vi "Central_Controller_SEF.vi"() -> ()   [LabVIEW 2019]
uses:
  <vilib>/Modbus/master/Modbus Master.lvclass
  C:/Program Files (x86)/National Instruments/LabVIEW 2019/vi.lib/Modbus/subvis/Modbus API/Modbus API.lvclass
  <vilib>/Modbus/subvis/Modbus API/Modbus API.lvclass/Modbus API.ctl
  <vilib>/Modbus/subvis/Transmission Data Unit (ADU)/Transmission Data Unit/Transmission Data Unit.lvclass/Transmission Data Unit.ctl
  <vilib>/Modbus/master/Data Access/Unit ID/Set Unit ID Property.vi
  <vilib>/Modbus/subvis/Transmission Data Unit (ADU)/Transmission Data Unit/Data Access/Unit ID/Write Unit ID.vi
  <vilib>/Modbus/subvis/Modbus API/Read Transmission Data Unit.vi
  <vilib>/Modbus/subvis/Modbus API/Write Transmission Data Unit.vi
  <vilib>/Modbus/master/Create Master Instance (TCP).vi
  <vilib>/Modbus/subvis/Transmission Data Unit (ADU)/Transmission Data Unit/Transmission Data Unit.lvclass
panel:
  out "Correct":bool
  out "Frequency":sgl
  out "SOLAR Real Power":sgl[](array[numeric])
  out "Array":errorcluster[](array[cluster])
  in  "Tab Control Islanding Extras":enum32{"Page 1"}(tab)
  in  "Relay 1 Num":u16
  in  "Relay 2 Num":u16
  in  "Relay 1":bool
  in  "Relay 2":bool
  in  "Tab Control Optimization Extras":enum32{"Page 1"}(tab)
  out "OPT Price":sgl[](array[numeric]) format="%#.3f"
  in  "OPT Alpha":sgl=0.1
  out "OPT Running No Error":bool
  out "In Range?":bool
  in  "Coerce":bool
  out "Attempts":i32
  in  "Reset Dual Variables":bool
  in  "Dispatch":bool
  in  "Array DER Index Dispatch":bool[](array[boolean])=[TRUE, TRUE, TRUE, TRUE, TRUE, TRUE, TRUE, TRUE, TRUE, TRUE, TRUE, TRUE, TRUE, FALSE, FALSE, TRUE]
  out "Pmax":sgl
  out "Pmin":sgl
  out "Pmin,i":sgl[](array[numeric])
  out "Pmax,i":sgl[](array[numeric])
  out "Indicator 15":sgl[](array[numeric])
  out "Indicator 14":sgl[](array[numeric])
  out "Indicator 13":sgl[](array[numeric])
  out "Indicator 12":sgl[](array[numeric])
  out "Indicator 11":sgl[](array[numeric])
  out "Indicator 10":sgl[](array[numeric])
  out "Indicator 9":sgl[](array[numeric])
  out "Indicator 8":sgl[](array[numeric])
  out "Indicator 7":sgl[](array[numeric])
  out "Indicator 6":sgl[](array[numeric])
  out "Indicator 5":sgl[](array[numeric])
  out "Indicator 4":sgl[](array[numeric])
  out "Indicator 3":sgl[](array[numeric])
  out "Indicator 2":sgl[](array[numeric])
  out "Indicator 1":sgl[](array[numeric])
  out "Indicator 0":sgl[](array[numeric])
  in  "DER List":string[](array[string])=["Capstone", "Aquion", "Tesla", "Load Bank", "Motor 1", "Simpliphi 1", "LG Chem", "Outback 1", "Outback 2", "Sunny Island", "ESS", "Fuel Cells", "Sparkplug", "Fronius", "Suny Boy", "Motor 2"]
  out "data":T1
  in  "File Name":string
  out "error out 3":errorcluster
  in  "Folder":path=path "C:/Users/administrator.STONEEDGEPOWER/Desktop/Data"
  out "Bid":sgl[](array[numeric])
  out "ALL Status":u16[](array[numeric])
  out "ALL AC RMS Line-Neutral Voltages":sgl[][](array[numeric])
  out "SYS Current Time":dbl format="%.3f"
  out "SYS DER Index":i32
  out "ALL Frequency":sgl[](array[numeric])
  out "ALL Control Method":string[](array[string])
  out "ALL Logged":bool[](array[boolean])
  out "ALL Through Variable":sgl[](array[numeric])
  out "ALL Across Variable":sgl[](array[numeric])
  out "ALL State of Charge":sgl[](array[numeric])
  out "ALL Reactive Power":sgl[](array[numeric])
  out "ALL Real Power":sgl[](array[numeric])
  out "ALL AC RMS Line-Line Average Voltage":sgl[][](array[numeric])
  in  "Tab Control Main":T2(tab)
  out "SYS H2 SoC":sgl format="%.1f"
  out "SYS H2 SoC Figure":sgl(slide) scale=0.0..100.0
  out "Free Power Flow Plot":sgl(graph)
  out "Free Power Flow Gauge":sgl(knob) caption="Gauge" scale=-100.0..100.0
  out "SYS SoC":sgl format="%.1f"
  out "SYS SoC Figure":sgl(slide) scale=0.0..100.0
  out "Free Power Flow":sgl
  out "DER0 Control Mode":string="Slave Mode Droops"
  out "LOAD Flow":i32(ring)
  out "LOAD Total Real Power":sgl format="%#.1f"
  out "DER13 Power Level":sgl format="%#.1f"
  out "DER14 Power Level":sgl format="%#.1f"
  out "DER13 Power Level Figure":sgl(slide)=1.0 scale=0.0..100.0
  out "DER3 State of Charge Figure":sgl(slide) scale=0.0..100.0
  out "DER3 State of Charge":sgl format="%.1f"
  out "DER0 Power Level Figure":sgl(slide)=1.0 scale=0.0..100.0
  out "DER14 Power Level Figure":sgl(slide)=1.0 scale=0.0..100.0
  out "SOLAR Flow":i32(ring)
  out "SOLAR Total Real Power":sgl format="%#.1f"
  out "DER15 Flow":i32(ring)
  out "DER14 Flow":i32(ring)
  out "DER13 Flow":i32(ring)
  out "DER12 Flow":i32(ring)
  out "DER5 Flow":i32(ring)
  out "DER4 Flow":i32(ring)
  out "DER3 Flow":i32(ring)
  out "DER1 Flow":i32(ring)
  out "DER0 Flow":i32(ring)
  in  "DER15 Detail Window Button":bool
  out "DER9 Reactive Power":sgl format="%.1f"
  out "DER10 State of Charge Figure":sgl(slide) scale=0.0..100.0
  out "DER10 State of Charge":sgl format="%#.1f"
  out "DER10 DC Voltage":sgl format="%.1f"
  out "PCC Meter":string
  in  "DER10 Detail Window Button":bool
  in  "DER13 Detail Window Button":bool
  in  "DER12 Detail Window Button":bool
  in  "DER2 Detail Window Button":bool
  in  "DER5 Detail Window Button":bool
  in  "DER9 Detail Window Button":bool
  in  "DER14 Detail Window Button":bool
  out "DER15 State of Charge Figure":sgl(slide) scale=0.0..100.0
  out "DER15 State of Charge":sgl format="%#.1f"
  out "DER15 Real Power":sgl format="%.1f"
  in  "DER15 Login Button":bool
  out "DER15 Logged":bool
  out "DER15 DC Voltage":sgl format="%#.1f"
  out "DER15 AC Line-Line Voltage":sgl=209.57935 format="%.1f"
  out "DER15 State":string
  in  "Island":bool
  out "DER8 State of Charge Figure":sgl(slide) scale=0.0..100.0
  out "DER8 State of Charge":sgl format="%#.1f"
  out "DER7 State of Charge Figure":sgl(slide) scale=0.0..100.0
  out "DER7 State of Charge":sgl format="%.1f"
  out "DER14 Real Power":sgl format="%.1f"
  in  "DER14 Login Button":bool
  out "DER14 Logged":bool
  out "DER14 DC Voltage":sgl format="%#.1f"
  out "DER14 AC Line-Line Voltage":sgl=209.57935 format="%.1f"
  out "DER9 State of Charge Figure":sgl(slide) scale=0.0..100.0
  out "DER9 Across Variable":sgl format="%.1g"
  out "DER9 State of Charge":sgl format="%.1f"
  out "DER13 AC Line-Line Voltage":sgl format="%.1f"
  out "DER13 Real Power":sgl format="%.1f"
  in  "DER13 Login Button":bool
  out "DER13 Logged":bool
  out "PCC Flow":i32(ring)
  out "DER8 DC Voltage":sgl format="%.1f"
  out "DER10 AC Line-Line Votlage":sgl format="%.1f"
  out "DER10 Real Power":sgl format="%.1f"
  in  "DER10 Login Button":bool
  out "DER10 Logged":bool
  out "DER7 Real Power":sgl format="%.1f"
  out "DER4 AC Line-Line Votlage":sgl format="%.1f"
  out "DER5 State of Charge Figure":sgl(slide) scale=0.0..100.0
  in  "DER0 Login Button":bool
  in  "DER2 Login Button":bool
  in  "DER1 Login Button":bool
  out "DER2 State of Charge Figure":sgl(slide) scale=0.0..100.0
  out "DER1 State of Charge Figure":sgl(slide) scale=0.0..100.0
  out "DER1 Real Power":sgl format="%.1f"
  out "DER1 Reactive Power":sgl format="%#.1f"
  out "DER1 AC Line-Line Voltage":sgl format="%.1f"
  out "DER2 Frequency":sgl format="%.1f"
  out "DER0 Real Power":sgl format="%#.1f"
  out "DER0 AC Line-Line Voltage":sgl format="%#.1f"
  out "DER2 AC Line-Line Voltage":sgl format="%.1f"
  out "DER2 Reactive Power":sgl format="%.1f"
  out "DER2 Real Power":sgl format="%.1f"
  out "DER0 Logged":bool
  out "DER1 Logged":bool
  out "DER2 Logged":bool
  out "DER0 Power Level":sgl format="%#.1f"
  out "DER1 State of Charge":sgl format="%.1f"
  out "DER2 State of Charge":sgl format="%#.1f"
  out "PCC Reactive Power":sgl
  out "PCC Real Power":sgl
  out "PCC AC Line-Line Voltage":sgl format="%#.1f"
  out "PCC Frequency":sgl format="%.2g"
  in  "DER3 Login Button":bool
  out "DER3 Logged":bool
  out "DER3 Real Power":sgl format="%#.1f"
  out "DER3 AC Line-Line Votlage":sgl format="%#.1f"
  out "DER4 State of Charge Figure":sgl(slide) scale=0.0..100.0
  out "DER4 State of Charge":sgl format="%#.1f"
  in  "DER4 Login Button":bool
  out "DER4 Logged":bool
  in  "DER5 Login Button":bool
  out "DER5 Across Variable":sgl format="%#.1f"
  out "DER5 logged":bool
  out "DER5 AC Line-Line Votlage":sgl format="%.1f"
  out "DER5 Real Power":sgl format="%.1f"
  out "PCC Real Power Duplicate":sgl format="%#_4g"
  in  "OPT Microgrid Set-point":sgl
  out "OPT Optimization Running Indicator":bool=TRUE
  in  "OPT Start Button":bool
  in  "OPT Stop Button":bool
  out "DER5 State of Charge":sgl format="%.1f"
  in  "DER7 Login Button":bool
  in  "DER8 Login Button":bool
  in  "DER9 Login Button":bool
  out "DER7 Logged":bool
  out "DER7 DC Voltage":sgl format="%.1g"
  out "DER7 AC Line-Line Voltage":sgl=209.57935 format="%.1f"
  out "DER8 AC Line-Line Votlage":sgl format="%.1f"
  out "DER8 Real Power":sgl format="%.1f"
  out "DER8 Logged":bool
  out "DER9 AC Line-Line Votlage":sgl format="%.1f"
  out "DER9 Real Power":sgl format="%.1f"
  out "DER9 Logged":bool
  out "DER12 AC Line-Line Votlage":sgl=209.57935 format="%.1f"
  out "DER12 DC Voltage":sgl format="%.1g"
  out "DER12 Logged":bool
  in  "DER12 Login Button":bool
  out "DER12 Real Power":sgl format="%.1g"
  out "DER4 Across Variable":sgl format="%#.1f"
  out "DER4 Real Power":sgl format="%#.1f"
  out "DER0 State":string
  out "DER1 State":string
  out "DER2 State":string
  out "DER3 State":string
  out "DER4 State":string
  out "DER5 State":string
  out "DER7 State":string
  out "DER8 State":string
  out "DER9 State":string
  out "DER10 State":string
  out "DER12 State":string
  out "DER13 State":string
  out "DER14 State":string
  in  "Reconnect":bool
  in  "DER0 Control Window Button":bool
  in  "DER0 Detail Window Button":bool
  in  "DER1 Detail Window Button":bool
  in  "DER1 Control Window Button":bool
  in  "DER2 Control Window Button":bool
  in  "DER3 Control Window Button":bool
  in  "DER4 Control Window Button":bool
  in  "DER5 Control Window Button":bool
  in  "DER7 Control Window Button":bool
  in  "DER8 Control Window Button":bool
  in  "DER9 Control Window Button":bool
  in  "DER10 Control Window Button":bool
  in  "DER12 Control Window Button":bool
  in  "DER13 Control Window Button":bool
  in  "DER14 Control Window Button":bool
  in  "DER15 Control Window Button":bool
  out "DER12 State of Charge":sgl format="%#.1f"
  out "DER12 State of Charge Figure":sgl(slide) scale=0.0..100.0
  in  "DER7 Detail Window Button":bool
  in  "DER3 Detail Window Button":bool
  in  "DER4 Detail Window Button":bool
  in  "DER8 Detail Window Button":bool
  out "DER2 Control Mode":string="Slave Mode Droops"
  out "DER14 Reactive Power":sgl format="%.1f"
  out "DER13 Reactive Power":sgl format="%.1f"
  out "DER1 Control Mode":string="Slave Mode Droops"
  out "DER2 Flow":i32(ring)
  out "DER7 Flow":i32(ring)
  out "DER8 Flow":i32(ring)
  out "DER9 Flow":i32(ring)
  out "DER10 Flow":i32(ring)
  out "PCC Real Power Figure":T3(graph)
  out "DER11 Flow":i32(ring)
  in  "DER11 Control Window Button":bool
  out "DER11 State":string
  out "DER11 AC Line-Line Votlage":sgl=209.57935 format="%.1f"
  out "DER11 Logged":bool
  in  "DER11 Login Button":bool
  out "DER11 Real Power":sgl format="%.1f"
  in  "DER11 Detail Window Button":bool
  out "DER11 Reactive Power":sgl format="%.1f"
  out "DER11 State of Charge":sgl format="%.1f"
  out "DER11 State of Charge Figure":sgl(slide) scale=0.0..100.0
  in  "DER6 Control Window Button":bool
  out "DER6 State":string
  out "DER6 AC Line-Line Voltage":sgl format="%.1f"
  out "DER6 Reactive Power":sgl format="%.1g"
  out "DER6 State of Charge":sgl format="%.1f"
  out "DER6 State of Charge Figure":sgl(slide) scale=0.0..100.0
  out "DER Logged":bool
  in  "DER6 Login Button":bool
  out "DER6 Real Power":sgl format="%.1g"
  in  "DER6 Detail Window Button":bool
  out "DER6 Flow":i32(ring)
  in  "Tab Control Communications":enum32{"Page 1"}(tab)
  in  "Enable Array":bool[](array[boolean])=[TRUE, FALSE, TRUE, FALSE, TRUE, TRUE, TRUE, FALSE, TRUE, TRUE, FALSE, FALSE, TRUE, TRUE, TRUE, TRUE]
  out "ALL Error Indicator":bool[](array[boolean])
  out "ALL DER Current Error":errorcluster[](array[cluster])
  out "ALL DER Final Error":errorcluster[](array[cluster])
  in  "PCC Meter IP Address":string[](array[string])=["10.0.1.53", "10.0.1.18"]
  out "PQM Current Error":errorcluster
  out "PQM Final Error":errorcluster
  in  "IP Address List":string[](array[string])=["10.0.1.182", "10.0.1.184", "10.0.1.180", "10.0.1.202", "10.0.1.189", "10.0.1.188", "10.0.1.190", "10.0.1.187", "10.0.1.195", "10.0.1.191", "10.0.1.185", "10.0.1.181", "10.0.1.201", "10.0.1.192", "10.0.1.207", "10.0.1.196"]
  in  "DERs Label Name":string[](array[string])=["DER0", "DER1", "DER2", "DER3", "DER4", "DER5", "DER6", "DER7", "DER8", "DER9", "DER10", "DER11", "DER12", "DER13", "DER14", "DER15"]
  out "Egauge Final Error":errorcluster
  out "Egauge Current Error":errorcluster
  out "SYS Iteration":i32
  in  "stop":bool
  out "SYS Status":string="Reading"
  out "SYS Case":i32
  in  "PCC Meter Label Name":string[](array[string])=["ASCO PQM", "Egauge"]
  in  "Solar Meter IP Address":string[](array[string])=["10.0.1.16"]
  in  "Solar Meter Label Name":string[](array[string])=["Solar 1 (Butler)", "Solar 2 (Agshed)", "Solar 3", "Solar 4", "Solar 5", "Solar 6"]
  out "PCC Meter Error Indicators":bool[](array[boolean])
  out "Solar Meter Error Indicators":bool[](array[boolean])
  # "DER0: Heila 2 , CAPSTONE, .182\nDER1: Heila 4, AQUION, .184\nDER2: Heila 0, TESLA, .180\nDER3: Heila 22, Load Bank, .202\nDER4: Heila 9, MOTOR 1, .189\nDER5: Heila 8, SIMPLIPHI 1, .188\nDER6: Heila 10, Solar Edge, .190\nDER7: Heila 7, OUTBACK 1, .187\nDER8: Heila15, OUTBACK 2, .195\nDER9: Heila 12, SUNNY ISLAND, .191\nDER10: Heila 5, ESS, .185\nDER11: Heila 1, Fuel Cells, .181\nDER12: Heila 21. Sparkplug, .201\nDER13: Heila 12, Fronius, .192\nDER14: Heila 27, Sunny Boy, .207\nDER15: Heila 16, Motor 2, .196"
  # "Islanding Extras"
  # "Optimization Extras"
  # "Consumption"
  # "Generation"
  # "Excess  Consumption"
  # "Excess Generation"
  # "Solar"
  # "Gas Turbine"
  # "HVAC"
  # "Loads"
  # "Battery"
  # "Hydrogen"
  # "SoC"
  # "%"
  # "SoC"
  # "%"
  # "Battery"
  # "Battery"
  # "Motor"
  # "Gas Turbine"
  # "Battery"
  # "Electrolyzer"
  # "Solar"
  # "Motor"
  # "Outback FLEX power"
  # "Capstone"
  # "Aquion + Ideal Power"
  # "Giner"
  # "LG + SolarEdge"
  # "LG + Sunny Boy"
  # "Hitachi VFD"
  # "Hitachi VFD"
  # "Status:"
  # "Status:"
  # "Status:"
  # "Status:"
  # "Status:"
  # "Status:"
  # "Status:"
  # "Status:"
  # "Mode:"
  # "Mode:"
  # "Solar"
  # "V"
  # "psi"
  # "V"
  # "psi"
  # "Real Microgrid in Real Time"
  # "SoC"
  # "%"
  # "SoC"
  # "SoC"
  # "%"
  # "SoC"
  # "%"
  # "p.u."
  # "%"
  # "%"
  # "SoC"
  # "%"
  # "p.u."
  # "%"
  # "SoC"
  # "%"
  # "kW"
  # "kW"
  # "kW"
  # "kW"
  # "kW"
  # "kW"
  # "kW"
  # "kW"
  # "Utility Grid"
  # "kW"
  # "V ="
  # "V"
  # "V"
  # "kVAr"
  # "V"
  # "V"
  # "kVAr"
  # "V"
  # "kVAr"
  # "V"
  # "f ="
  # "Hz"
  # "PG&E"
  # "P ="
  # "W"
  # "V"
  # "V"
  # "V"
  # "Q ="
  # "VAr"
  # "Optimization:"
  # "kW"
  # "kW"
  # "kW"
  # "kVAr"
  # "kW"
  # "kW"
  # "PCC Set-point:"
  # "kW"
  # "kW"
  # "kW"
  # "kW"
  # "V"
  # "kVAr"
  # "kVAr"
  # "kW"
  # "kVAr"
  # "V"
  # "V"
  # "V"
  # "V"
  # "V"
  # "V"
  # "V"
  # "Hz"
  # "PCC Power:"
  # "kW"
  # "Battery"
  # "Battery"
  # "Fuel Cells"
  # "Battery"
  # "Battery"
  # "Battery"
  # "Battery"
  # "Solar"
  # "Load"
  # "Sony + Outback"
  # "Relion"
  # "Simpliphi + SMA"
  # "Tesla + Dynapower"
  # "Simpliphi + Schneider"
  # "Simpliphi + Schneider"
  # "LG + Fronius"
  # "ESS"
  # "Status:"
  # "Status:"
  # "Status:"
  # "Status:"
  # "Status:"
  # "Status:"
  # "Status:"
  # "Status:"
  # "Mode:"
  # "V"
  # "V"
  # "V"
  # "V"
  # "V"
  # "SoC"
  # "%"
  # "SoC"
  # "%"
  # "SoC"
  # "%"
  # "SoC"
  # "%"
  # "SoC"
  # "%"
  # "SoC"
  # "%"
  # "SoC"
  # "%"
  # "p.u."
  # "%"
  # "Reading from:"
  # "Program"
  # "Controllable DERs"
  # "PCC Meters"
  # "Solar Array Meters"
  # "DER0: Heila 2 , CAPSTONE, .182\nDER1: Heila 4, AQUION, .184\nDER2: Heila 0, TESLA, .180\nDER3: Heila 22, Load Bank, .202\nDER4: Heila 9, MOTOR 1, .189\nDER5: Heila 8, SIMPLIPHI 1, .188\nDER6: Heila 10, Solar Edge, .190\nDER7: Heila 7, OUTBACK 1, .187\nDER8: Heila15, OUTBACK 2, .195\nDER9: Heila 12, SUNNY ISLAND, .191\nDER10: Heila 5, ESS, .185\nDER11: Heila 1, Fuel Cells, .181\nDER12: Heila 21. Sparkplug, .201\nDER13: Heila 12, Fronius, .192\nDER14: Heila 27, Sunny Boy, .207\nDER15: Heila 16, Motor 2, .196"
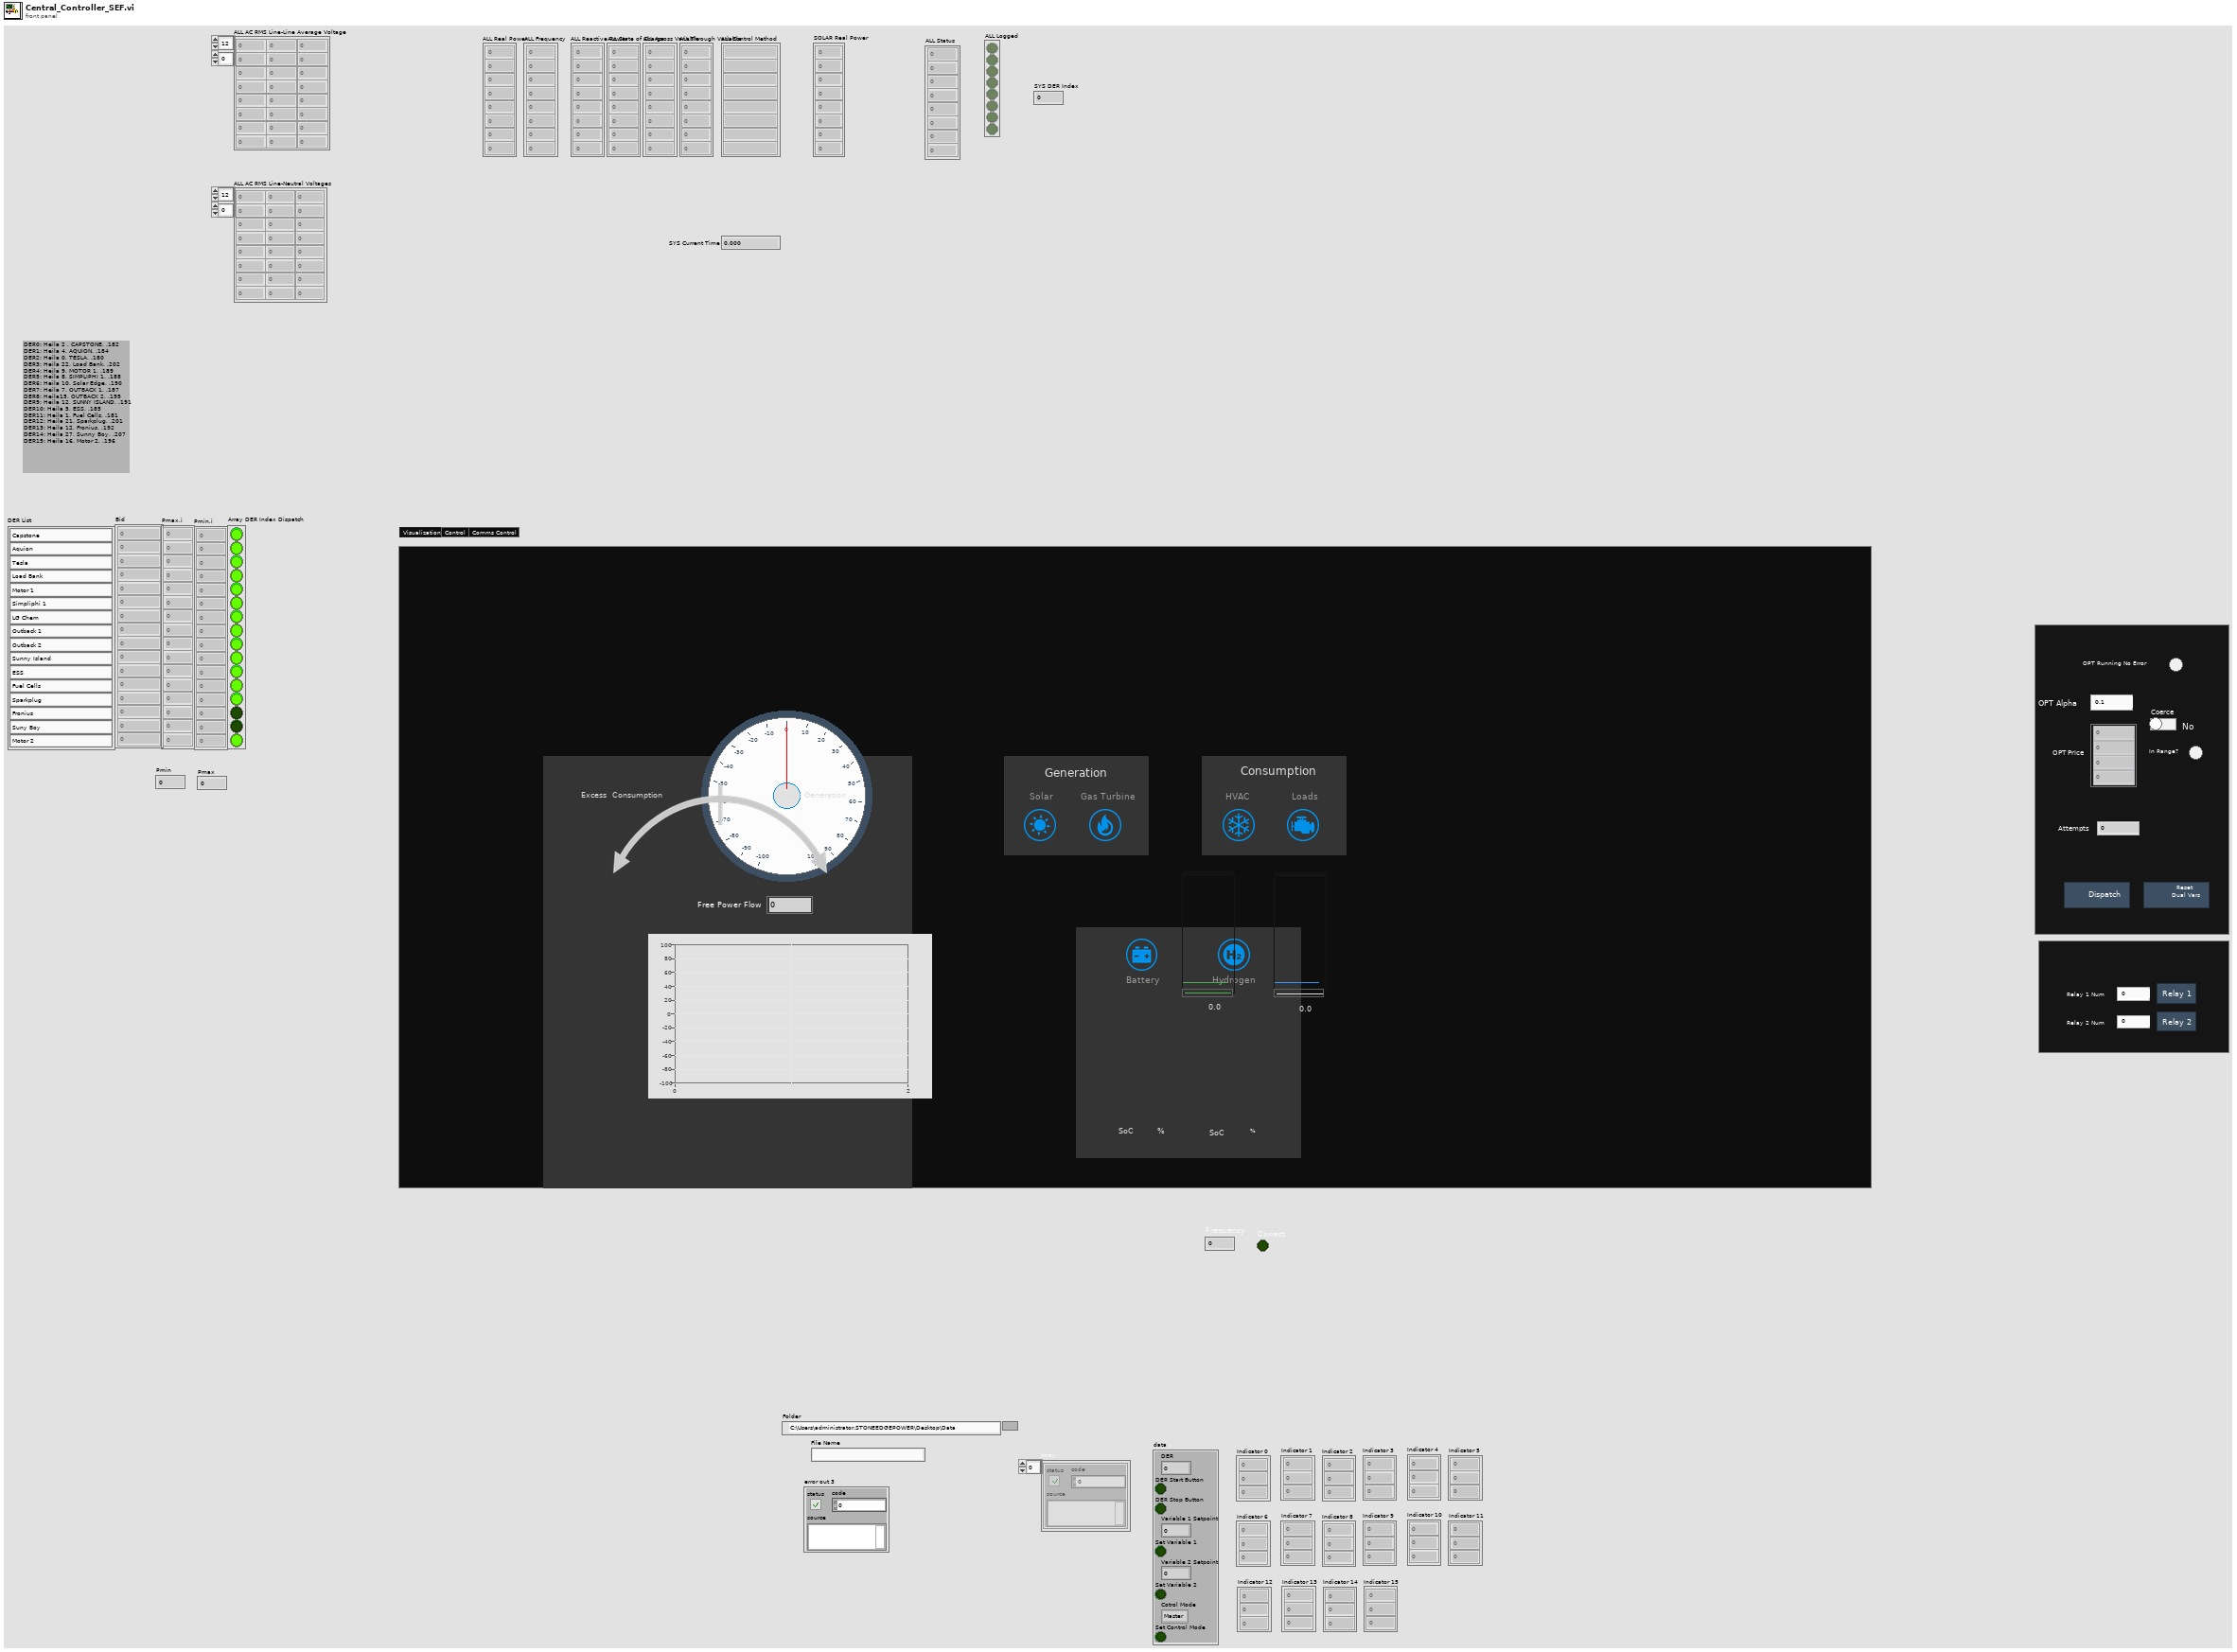
[diagram p1: front panel]
types:
  T1 = cluster{"DER":i32, "DER Start Button":bool, "DER Stop Button":bool, "Variable 1 Setpoint":sgl, "Set Variable 1":bool, "Variable 2 Setpoint":sgl, "Set Variable 2":bool, "Cotrol Mode":enum16{"Master", "Slave"}, "Set Control Mode":bool}
  T2 = enum32{"Visualization", "Control", "Comms Control"}
  T3 = cluster{"[0]":sgl, "[1]":sgl, "[2]":sgl, "[3]":sgl, "[4]":sgl}
  T4 = enum16{"open", "replace", "create", "open or create", "replace or create", "replace or create with confirmation"}
  T5 = cluster{"Modbus master out":refnum<class "Modbus Master.lvclass">, "error out":errorcluster}[]
  T6 = cluster{"Modbus master out":refnum<class "Modbus Master.lvclass">, "error out":errorcluster}
  T7 = enum32{"Invalid", "Standard", "Closed", "Hidden", "Minimized", "Maximized"}
  T8 = cluster{"Modbus master out":refnum<class "Modbus Master.lvclass">, "error IO":errorcluster}
  T9 = enum32{"Bad", "Idle", "Run top level", "Running"}
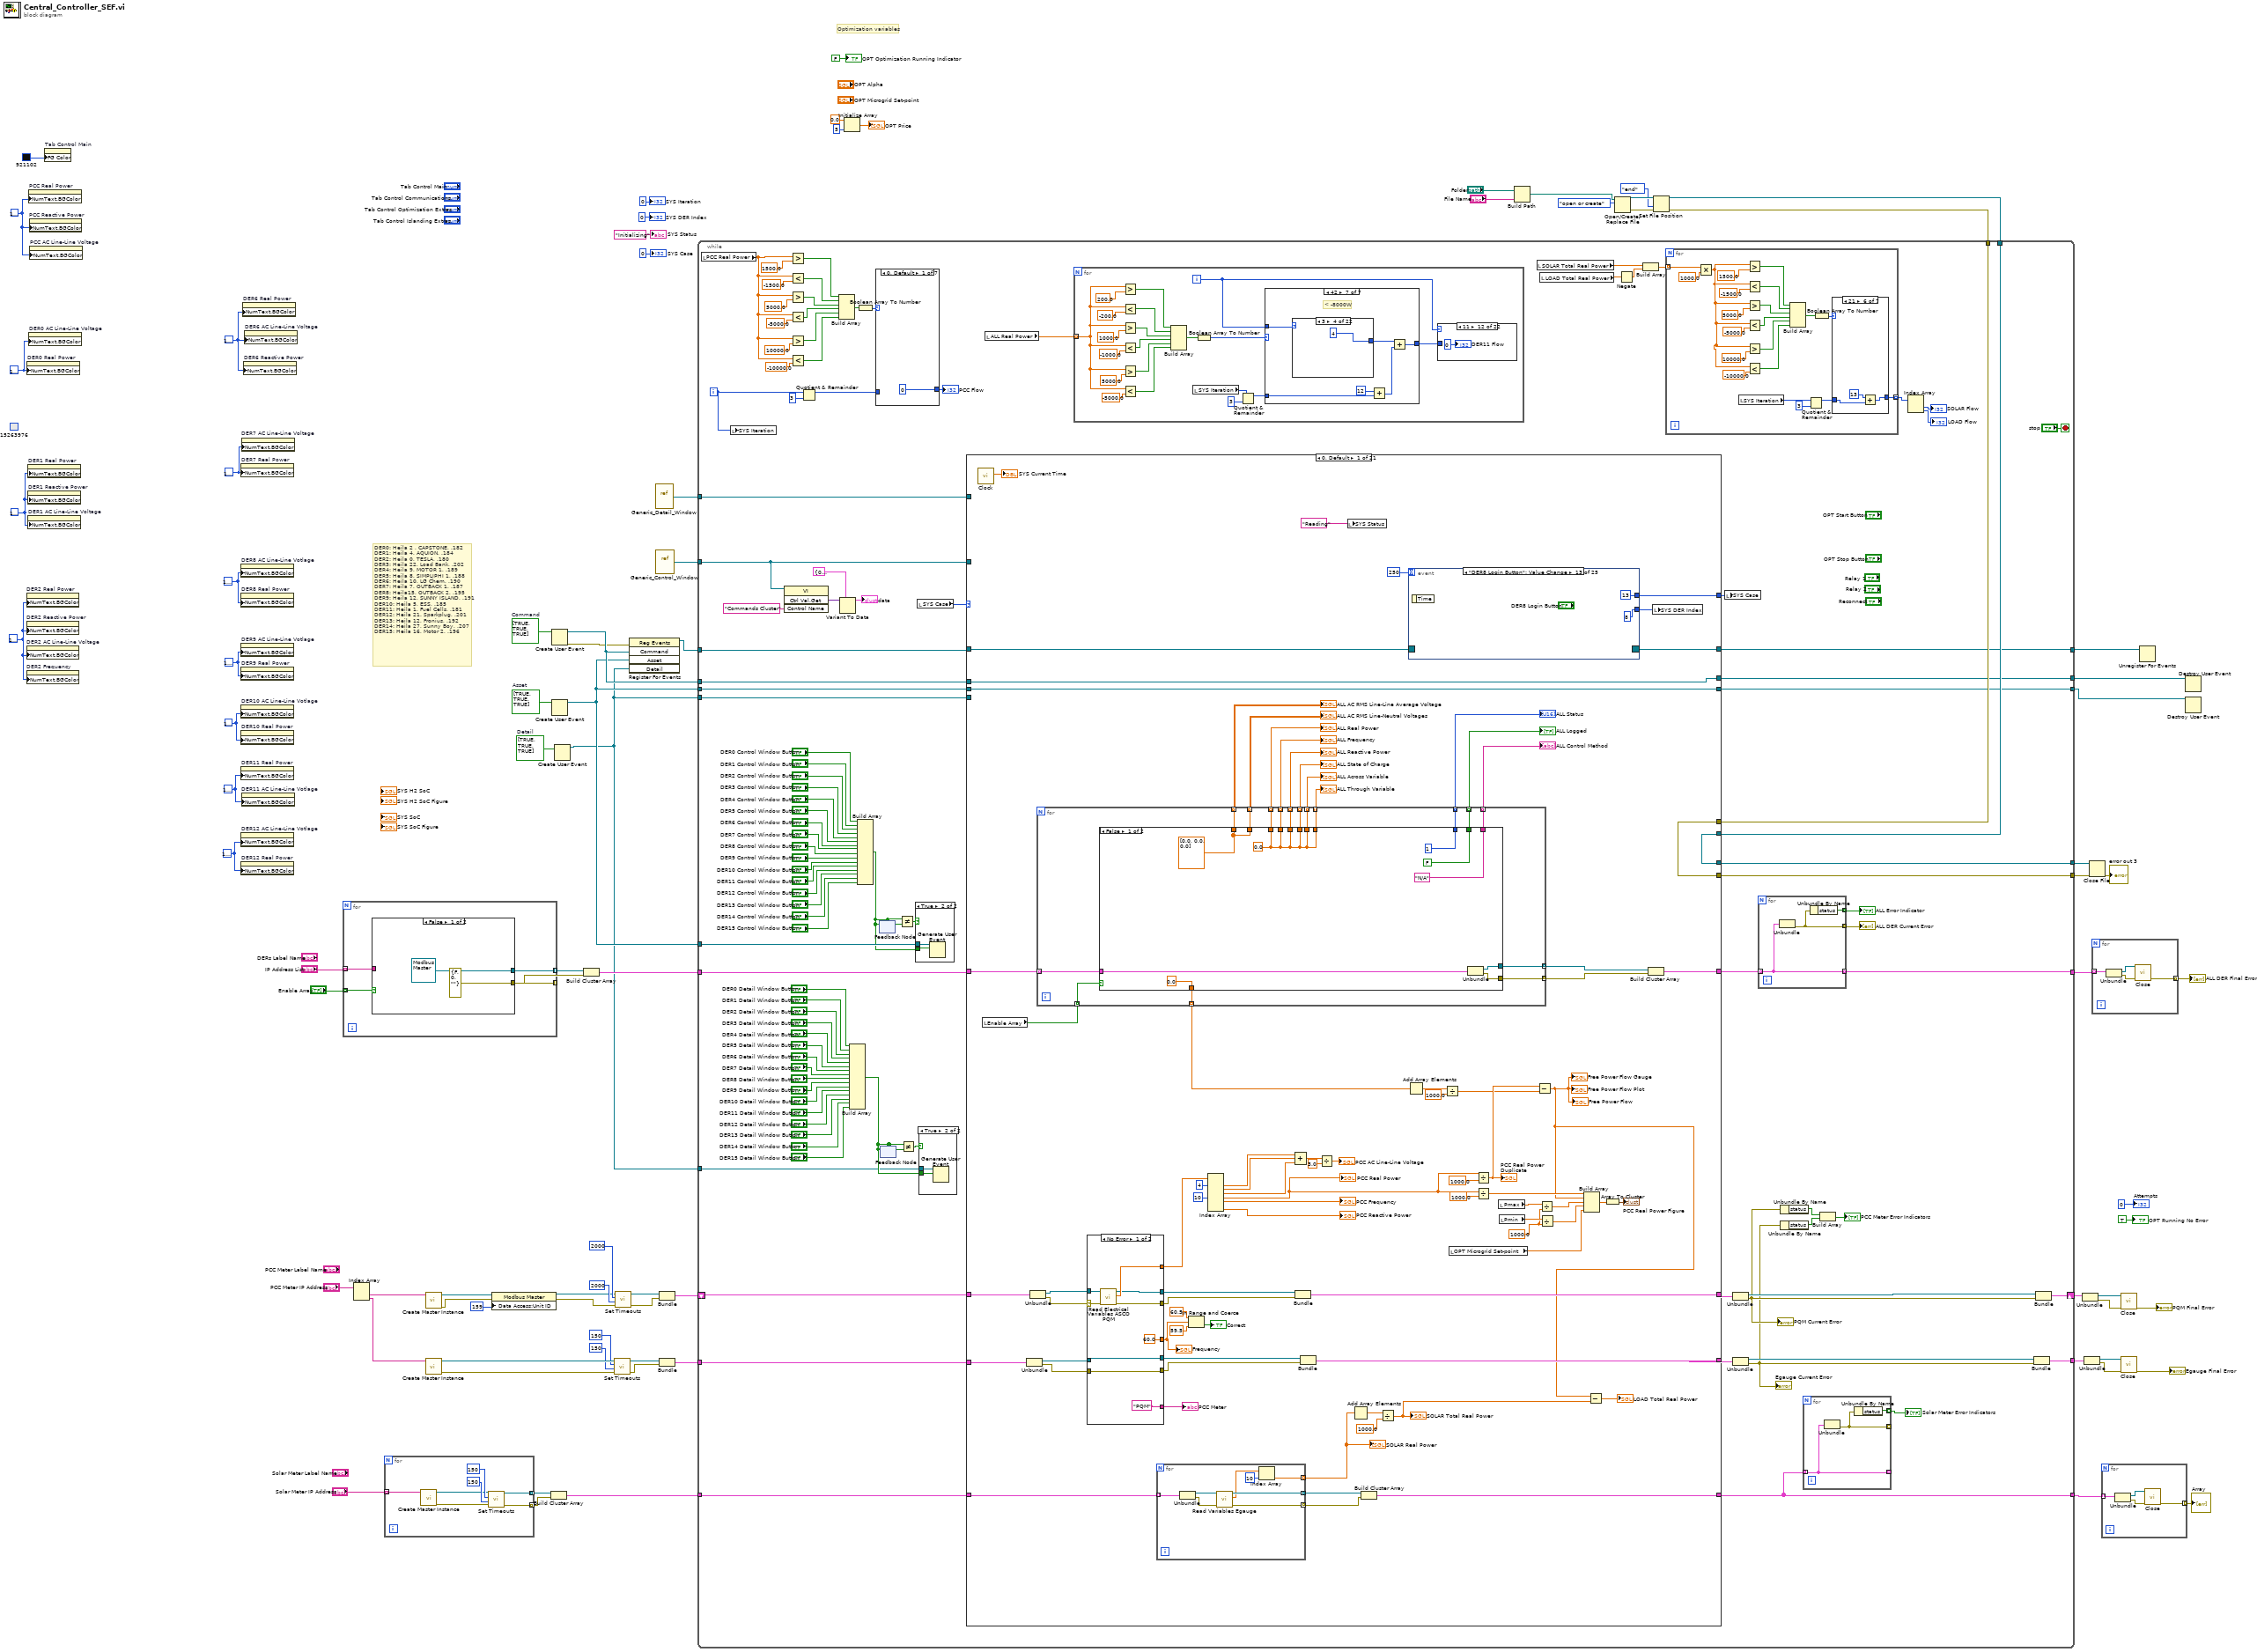
[diagram p0: block diagram]
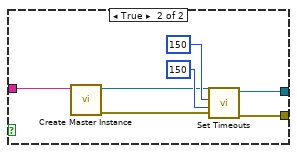
[diagram p2: hidden frame]
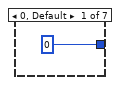
[diagram p3: hidden frame]
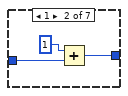
[diagram p4: hidden frame]
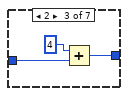
[diagram p5: hidden frame]
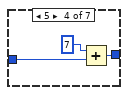
[diagram p6: hidden frame]
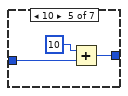
[diagram p7: hidden frame]
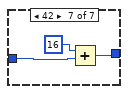
[diagram p8: hidden frame]
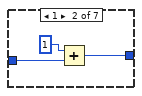
[diagram p11: hidden frame]
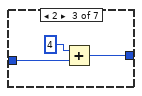
[diagram p12: hidden frame]
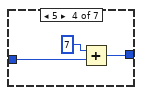
[diagram p13: hidden frame]
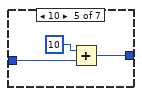
[diagram p14: hidden frame]
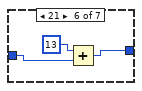
[diagram p15: hidden frame]
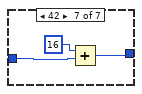
[diagram p16: hidden frame]
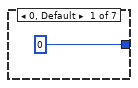
[diagram p17: hidden frame]
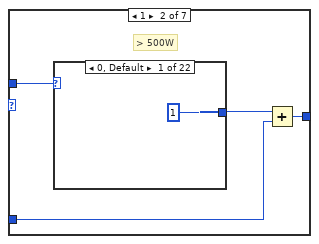
[diagram p18: hidden frame]
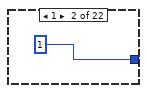
[diagram p19: hidden frame]
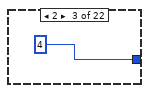
[diagram p20: hidden frame]
diagram:
  w4 = bool[] [TRUE, TRUE, TRUE]  # Detail
  w36 = bool[] [TRUE, TRUE, TRUE]  # Asset
  w39 = bool[] [TRUE, TRUE, TRUE]  # Command
  w57 = u32 16777216
  w56 = u32 16777216
  w60 = u32 16777216
  w59 = u32 16777216
  w58 = u32 16777216
  w61 = u32 16777216
  w62 = u32 16777216
  w79 = u32 16777216
  w84 = u32 16777216
  w85 = u32 16777216
  w86 = u32 16777216
  (unwired) u32 15263976
  # "DER0: Heila 2 , CAPSTONE, .182\nDER1: Heila 4, AQUION, .184\nDER2: Heila 0, TESLA, .180\nDER3: Heila 22, Load Bank, .202\nDER4: Heila 9, MOTOR 1, .189\nDER5: Heila 8, SIMPLIPHI 1, .188\nDER6: Heila 10, LG Chem, .190\nDER7: Heila 7, OUTBACK 1, .187\nDER8: Heila15, OUTBACK 2, .195\nDER9: Heila 12, SUNNY ISLAND, .191\nDER10: Heila 5, ESS, .185\nDER11: Heila 1, Fuel Cells, .181\nDER12: Heila 21. Sparkplug, .201\nDER13: Heila 12, Fronius, .192\nDER14: Heila 27, Sunny Boy, .207\nDER15: Heila 16, Motor 2, .196"
  # "Optimization variables"
  n1 = property on="DER2 Real Power" class="DigNum (strict)"("NumText.BGColor"=w84) -> ()  [unwired: 2 in, 2 out]
  n2 = property on="DER2 Reactive Power" class="DigNum (strict)"("NumText.BGColor"=w84) -> ()  [unwired: 2 in, 2 out]
  n3 = property on="DER2 AC Line-Line Voltage" class="DigNum (strict)"("NumText.BGColor"=w84) -> ()  [unwired: 2 in, 2 out]
  n4 = property on="DER2 Frequency" class="DigNum (strict)"("NumText.BGColor"=w84) -> ()  [unwired: 2 in, 2 out]
  n5 = property on="DER0 Real Power" class="DigNum (strict)"("NumText.BGColor"=w86) -> ()  [unwired: 2 in, 2 out]
  n6 = property on="DER1 Real Power" class="DigNum (strict)"("NumText.BGColor"=w85) -> ()  [unwired: 2 in, 2 out]
  n7 = property on="DER1 Reactive Power" class="DigNum (strict)"("NumText.BGColor"=w85) -> ()  [unwired: 2 in, 2 out]
  n8 = property on="DER1 AC Line-Line Voltage" class="DigNum (strict)"("NumText.BGColor"=w85) -> ()  [unwired: 2 in, 2 out]
  n9 = property on="PCC Real Power" class="DigNum (strict)"("NumText.BGColor"=w79) -> ()  [unwired: 2 in, 2 out]
  n10 = property on="DER0 AC Line-Line Voltage" class="DigNum (strict)"("NumText.BGColor"=w86) -> ()  [unwired: 2 in, 2 out]
  n11 = property on="PCC Reactive Power" class="DigNum (strict)"("NumText.BGColor"=w79) -> ()  [unwired: 2 in, 2 out]
  n12 = property on="PCC AC Line-Line Voltage" class="DigNum (strict)"("NumText.BGColor"=w79) -> ()  [unwired: 2 in, 2 out]
  n13 = property on="Tab Control Main" class="TabCtl (strict)"("FG Color"=u32 921102) -> ()  [unwired: 2 in, 2 out]
  n14 = property on="DER7 Real Power" class="DigNum (strict)"("NumText.BGColor"=w61) -> ()  [unwired: 2 in, 2 out]
  n15 = property on="DER8 AC Line-Line Votlage" class="DigNum (strict)"("NumText.BGColor"=w58) -> ()  [unwired: 2 in, 2 out]
  n16 = property on="DER8 Real Power" class="DigNum (strict)"("NumText.BGColor"=w58) -> ()  [unwired: 2 in, 2 out]
  n17 = property on="DER9 AC Line-Line Votlage" class="DigNum (strict)"("NumText.BGColor"=w59) -> ()  [unwired: 2 in, 2 out]
  n18 = property on="DER9 Real Power" class="DigNum (strict)"("NumText.BGColor"=w59) -> ()  [unwired: 2 in, 2 out]
  n19 = property on="DER10 AC Line-Line Votlage" class="DigNum (strict)"("NumText.BGColor"=w60) -> ()  [unwired: 2 in, 2 out]
  n20 = property on="DER10 Real Power" class="DigNum (strict)"("NumText.BGColor"=w60) -> ()  [unwired: 2 in, 2 out]
  n21 = property on="DER11 Real Power" class="DigNum (strict)"("NumText.BGColor"=w56) -> ()  [unwired: 2 in, 2 out]
  n22 = property on="DER12 AC Line-Line Votlage" class="DigNum (strict)"("NumText.BGColor"=w57) -> ()  [unwired: 2 in, 2 out]
  n23 = property on="DER12 Real Power" class="DigNum (strict)"("NumText.BGColor"=w57) -> ()  [unwired: 2 in, 2 out]
  n24 = property on="DER7 AC Line-Line Voltage" class="DigNum (strict)"("NumText.BGColor"=w61) -> ()  [unwired: 2 in, 2 out]
  n25 = property on="DER11 AC Line-Line Votlage" class="DigNum (strict)"("NumText.BGColor"=w56) -> ()  [unwired: 2 in, 2 out]
  n26 = property on="DER6 Real Power" class="DigNum (strict)"("NumText.BGColor"=w62) -> ()  [unwired: 2 in, 2 out]
  n27 = property on="DER6 Reactive Power" class="DigNum (strict)"("NumText.BGColor"=w62) -> ()  [unwired: 2 in, 2 out]
  n28 = property on="DER6 AC Line-Line Voltage" class="DigNum (strict)"("NumText.BGColor"=w62) -> ()  [unwired: 2 in, 2 out]
  n29 = for {
    tunnel: "IP Address List" -> [w92] mode=indexing
    tunnel: [w91] -> w77 mode=indexing
    tunnel: [w90] -> w76 mode=indexing
    tunnel: "Enable Array" -> [w89] mode=indexing
    n30 = case shown="False" w89 {
      tunnel: w92 -> [_ w101]
      tunnel: [refnum<class "Modbus Master.lvclass"> refnum ("Modbus master out") w98] -> w91
      tunnel: [errorcluster {"status"=FALSE, "code"=0, "source"=""} ("error out") w97] -> w90
      frame False {
      }
      frame True {
        n31 = call-poly <vilib>:"Create Master Instance.vi"("address"=w101) -> ("error out"=w95:errorcluster, "TCP master instance"=w96:refnum<class "Modbus Master.lvclass">)  [unwired: 9 in]
        n32 = call <vilib>:"Set Timeouts.vi"("error in (no error)"=w95, "write operation timeout (ms)"=150 ("Write Timeout"), "read operation timeout (ms)"=150 ("Read Timeout"), "Modbus master in"=w96) -> ("error out"=w97:errorcluster, "Modbus master out"=w98:refnum<class "Modbus Master.lvclass">)  [unwired: 6 in]
      }
    }
  }
  n33 = Index Array(array="PCC Meter IP Address") -> (element #1=w12:string, element #2=w11:string)  [unwired: 2 in]
  n34 = for {
    tunnel: "Solar Meter IP Address" -> [w108] mode=indexing
    tunnel: [w103] -> w9 mode=indexing
    tunnel: [w102] -> w8 mode=indexing
    n35 = call-poly <vilib>:"Create Master Instance.vi"("address"=w108) -> ("error out"=w104:errorcluster, "TCP master instance"=w105:refnum<class "Modbus Master.lvclass">)  [unwired: 9 in]
    n36 = call <vilib>:"Set Timeouts.vi"("error in (no error)"=w104, "write operation timeout (ms)"=150 ("Write Timeout"), "read operation timeout (ms)"=150 ("Read Timeout"), "Modbus master in"=w105) -> ("error out"=w102:errorcluster, "Modbus master out"=w103:refnum<class "Modbus Master.lvclass">)  [unwired: 6 in]
  }
  n37 = call-poly <vilib>:"Create Master Instance.vi"("address"=w12) -> ("error out"=w80:errorcluster, "TCP master instance"=w81:refnum<class "Modbus Master.lvclass">)  [unwired: 9 in]
  n38 = call-poly <vilib>:"Create Master Instance.vi"("address"=w11) -> ("error out"=w28:errorcluster, "TCP master instance"=w29:refnum<class "Modbus Master.lvclass">)  [unwired: 9 in]
  n39 = property class="Modbus Master"(reference=w81, error in=w80, "Data Access:Unit ID"=u8 159 ("Unit ID")) -> (reference out=w64:refnum<class "Modbus Master.lvclass">, error out=w63:errorcluster)
  n40 = Build Cluster Array(w9, w8) -> (w7:T5)
  n41 = Create User Event(user event datatype=w39) -> (user event=w37:refnum<user-event>, error out=w33:errorcluster)  [unwired: 1 in]
  n42 = Create User Event(user event datatype=w36) -> (user event=w32:refnum<user-event>)  [unwired: 1 in, 1 out]
  n43 = Create User Event(user event datatype=w4) -> (user event=w2:refnum<user-event>)  [unwired: 1 in, 1 out]
  n44 = Build Cluster Array(w77, w76) -> (w75:T5)
  n45 = call <vilib>:"Set Timeouts.vi"("error in (no error)"=w28, "write operation timeout (ms)"=150 ("Write Timeout"), "read operation timeout (ms)"=150 ("Read Timeout"), "Modbus master in"=w29) -> ("error out"=w24:errorcluster, "Modbus master out"=w25:refnum<class "Modbus Master.lvclass">)  [unwired: 6 in]
  n46 = call <vilib>:"Set Timeouts.vi"("error in (no error)"=w63, "write operation timeout (ms)"=2000 ("Write Timeout"), "read operation timeout (ms)"=2000 ("Read Timeout"), "Modbus master in"=w64) -> ("error out"=w18:errorcluster, "Modbus master out"=w19:refnum<class "Modbus Master.lvclass">)  [unwired: 6 in]
  n47 = register-events(error in=w33, w37, w32, w2) -> (reference out=w38:refnum<event-registration>)  [unwired: 1 in, 1 out]
  n48 = vi-ref "Generic_Detail_Window.vi"() -> (w3:refnum<vi>)
  n49 = vi-ref "Generic_Control_Window.vi"() -> (w40:refnum<vi>)
  n50 = Bundle("Modbus master out"=w19, "error out"=w18) -> (w14:T6)  [unwired: 1 in]
  n51 = Bundle("Modbus master out"=w25, "error out"=w24) -> (w23:T6)  [unwired: 1 in]
  n52 = Initialize Array(sgl 0.0 ("element"), 5 ("dimension size")) -> (→"OPT Price":sgl[])
  n53 = Build Path(base path="Folder", name or relative path="File Name") -> (appended path=w41:path)
  n54 = Open/Create/Replace File(file path (use dialog)=w41, operation (0:open)=T4."open or create") -> (refnum out=w51:refnum<file>, error out=w50:errorcluster)  [unwired: 4 in, 1 out]
  n55 = Set File Position(refnum=w51, from (0:start)=enum16{"start", "end", "current"}."end", error in=w50) -> (refnum out=w45:refnum<file>, error out=w44:errorcluster)  [unwired: 1 in]
  n56 = while {
    tunnel: w75 -> [w213]
    tunnel: [w209] -> w67
    tunnel: [w203] -> w48
    tunnel: [w202] -> w47
    tunnel: w45 -> [w201]
    tunnel: w44 -> [w200]
    tunnel: w40 -> [w169]
    tunnel: w37 -> [w198]
    tunnel: w32 -> [w189]
    tunnel: [w185] -> w34
    tunnel: w32 -> [w184]
    tunnel: [w183] -> w31
    tunnel: w38 -> [w199]
    tunnel: [w186] -> w35
    tunnel: w23 -> [w167]
    tunnel: [w164] -> w20
    shift-right: [w161] -> w17
    shift-left: w14 -> [w163]
    tunnel: w7 -> [w160]
    tunnel: [w154] -> w6
    tunnel: w2 -> [w118]
    tunnel: w3 -> [w117]
    tunnel: w2 -> [w116]
    i -> [w207]
    stop <- "stop" stop-if-true
    n57 = local read "PCC Real Power"() -> (w138:sgl)
    n58 = local write "SYS Iteration"(w207) -> ()
    n59 = invoke class="VI" method="Ctrl Val.Get"(reference=w169, "Control Name"="Commands Cluster") -> ("Get Control Value Variant"=w197:variant)  [unwired: 2 in, 3 out]
    n60 = Greater?(x=w138, y=sgl 1500.0) -> (0:w149:bool)
    n61 = Less?(x=w138, y=sgl -1500.0) -> (x < y?=w148:bool)
    n62 = Greater?(x=w138, y=sgl 5000.0) -> (0:w143:bool)
    n63 = Less?(x=w138, y=sgl -5000.0) -> (x < y?=w142:bool)
    n64 = Greater?(x=w138, y=sgl 10000.0) -> (0:w141:bool)
    n65 = Less?(x=w138, y=sgl -10000.0) -> (x < y?=w140:bool)
    n66 = Quotient & Remainder(x=w207, y=3) -> (x-y*floor(x/y)=w206:i32)  [unwired: 1 out]
    n67 = Build Array(w149, w148, w143, w142, w141, w140) -> (w139:bool[])
    n68 = Variant To Data(type=T1 {"DER"=0, "DER Start Button"=FALSE, "DER Stop Button"=FALSE, "Variable 1 Setpoint"=0.0, "Set Variable 1"=FALSE, "Variable 2 Setpoint"=0.0, "Set Variable 2"=FALSE, "Cotrol Mode"=enum."Slave", "Set Control Mode"=FALSE} ("Commands Cluster 2"), Variant=w197) -> (data=→"data":T1)  [unwired: 1 in, 1 out]
    n69 = Build Array("DER0 Detail Window Button", "DER1 Detail Window Button", "DER2 Detail Window Button", "DER3 Detail Window Button", "DER4 Detail Window Button", "DER5 Detail Window Button", "DER6 Detail Window Button", "DER7 Detail Window Button", "DER8 Detail Window Button", "DER9 Detail Window Button", "DER10 Detail Window Button", "DER11 Detail Window Button", "DER12 Detail Window Button", "DER13 Detail Window Button", "DER14 Detail Window Button", "DER15 Detail Window Button") -> (w120:bool[])
    n70 = Boolean Array To Number(Boolean array=w139) -> (number=w204:u32)
    n71 = Build Array("DER0 Control Window Button", "DER1 Control Window Button", "DER2 Control Window Button", "DER3 Control Window Button", "DER4 Control Window Button", "DER5 Control Window Button", "DER6 Control Window Button", "DER7 Control Window Button", "DER8 Control Window Button", "DER9 Control Window Button", "DER10 Control Window Button", "DER11 Control Window Button", "DER12 Control Window Button", "DER13 Control Window Button", "DER14 Control Window Button", "DER15 Control Window Button") -> (w188:bool[])
    n72 = case shown="0, Default" w204 {
      tunnel: [0 w266 w269 w272 w275 w278 w281] -> w152
      tunnel: w206 -> [_ w265 w268 w271 w274 w277 w280]
      frame 0, Default {
      }
      frame 1 {
        n73 = Add(x=1, y=w265) -> (x+y=w266:i32)
      }
      frame 2 {
        n74 = Add(x=4, y=w268) -> (x+y=w269:i32)
      }
      frame 5 {
        n75 = Add(x=7, y=w271) -> (x+y=w272:i32)
      }
      frame 10 {
        n76 = Add(x=10, y=w274) -> (x+y=w275:i32)
      }
      frame 21 {
        n77 = Add(x=13, y=w277) -> (x+y=w278:i32)
      }
      frame 42 {
        n78 = Add(x=16, y=w280) -> (x+y=w281:i32)
      }
    }
    "PCC Flow" <- w152
    n79 = feedback-in #1(w188) -> ()
    n80 = feedback #1(w188) -> (w190:bool[])
    n81 = feedback #2(w120) -> (w121:bool[])
    n82 = feedback-in #2(w120) -> ()
    n83 = Not Equal?(x=w188, y=w190) -> (x != y?=w182:bool)
    n84 = Not Equal?(x=w120, y=w121) -> (x != y?=w119:bool)
    n85 = case shown="True" w182 {
      tunnel: w189 -> [_ w263]
      tunnel: w188 -> [_ w262]
      frame False {
      }
      frame True {
        n86 = Generate User Event(user event=w263, event data cluster=w262) -> ()  [unwired: 2 in, 2 out]
      }
    }
    n87 = local read "SYS Case"() -> (w215:i32)
    n88 = case shown="True" w119 {
      tunnel: w118 -> [_ w258]
      tunnel: w120 -> [_ w257]
      frame False {
      }
      frame True {
        n89 = Generate User Event(user event=w258, event data cluster=w257) -> ()  [unwired: 2 in, 2 out]
      }
    }
    n90 = case shown="0, Default" w215 {
      tunnel: [w567 2 w1002 0 0 0 0 0 0 0 0 0 0 0 0 0 0 0 0 w1423 w1456] -> w168
      tunnel: [w520 w732 w980 w1008 w1025 w1042 w1072 w1095 w1117 w1139 w1192 w1216 w1233 w1251 w1277 w1303 w1329 w1355 w1403 w1421 w1454] -> w214
      tunnel: w163 -> [w552 w732 w980 w1008 w1025 w1042 w1072 w1095 w1117 w1139 w1192 w1216 w1233 w1258 w1284 w1310 w1336 w1368 w1403 w1421 w1454]
      tunnel: [w562 w746 w999 w1012 w1029 w1049 w1085 w1101 w1122 w1144 w1182 w1220 w1236 w1260 w1286 w1312 w1338 w1370 w1407 w1427 w1458] -> w212
      tunnel: w213 -> [w565 w746 w999 w1014 w1030 w1053 w1086 w1100 w1123 w1145 w1195 w1223 w1237 w1260 w1286 w1312 w1338 w1370 w1408 w1427 w1458]
      tunnel: [w536 _ w992 _ _ _ _ _ _ _ _ _ _ _ _ _ _ _ _ _ _] -> w203
      tunnel: [w537 _ w991 _ _ _ _ _ _ _ _ _ _ _ _ _ _ _ _ _ _] -> w202
      tunnel: w201 -> [w536 _ w990 _ _ _ _ _ _ _ _ _ _ _ _ _ _ _ _ _ _]
      tunnel: w200 -> [w537 _ w989 _ _ _ _ _ _ _ _ _ _ _ _ _ _ _ _ _ _]
      tunnel: w169 -> [_ _ _ _ _ _ _ _ _ _ _ _ _ _ _ _ _ _ _ w1424 _]
      tunnel: w199 -> [w535 w734 w982 _ _ _ _ _ _ _ _ _ _ _ _ _ _ _ _ _ _]
      tunnel: [w534 w734 w982 _ _ _ _ _ _ _ _ _ _ _ _ _ _ _ _ _ _] -> w186
      tunnel: w198 -> [w533 _ _ _ _ _ _ _ _ _ _ _ _ _ _ _ _ _ _ w1426 _]
      tunnel: [w533 _ _ _ _ _ _ _ _ _ _ _ _ _ _ _ _ _ _ _ _] -> w185
      tunnel: w184 -> [w532 _ _ _ _ _ _ _ _ _ _ _ _ _ _ _ _ _ _ _ _]
      tunnel: [w532 _ _ _ _ _ _ _ _ _ _ _ _ _ _ _ _ _ _ _ _] -> w183
      tunnel: w167 -> [w527 w733 w981 w1009 w1026 w1043 w1073 w1096 w1118 w1140 w1193 w1217 w1234 w1250 w1276 w1302 w1328 w1354 w1404 w1422 w1455]
      tunnel: [w526 w733 w981 w1009 w1026 w1043 w1073 w1096 w1118 w1140 w1193 w1217 w1234 w1250 w1276 w1302 w1328 w1354 w1404 w1422 w1455] -> w166
      tunnel: w160 -> [w502 w731 w978 w1007 w1024 w1041 w1071 w1094 w1116 w1138 w1160 w1215 w1232 w1249 w1275 w1301 w1327 w1353 w1401 w1420 w1453]
      tunnel: [w499 w731 w978 w1007 w1024 w1041 w1071 w1094 w1116 w1138 w1160 w1215 w1232 w1249 w1275 w1301 w1327 w1353 w1401 w1420 w1453] -> w154
      tunnel: w117 -> [_ _ _ _ _ _ _ _ _ _ _ _ _ _ _ _ _ _ _ _ w1452]
      tunnel: w116 -> [_ _ _ _ _ _ _ _ _ _ _ _ _ _ _ _ _ _ _ _ _]
      frame 0, Default {
        w505 = sgl 1000.0
        n91 = call "Clock.vi"() -> ("SYS Current Time"=→"SYS Current Time":dbl)  [unwired: 11 in]
        n92 = local read "Enable Array"() -> (w488:bool[])
        n93 = Unbundle(w527) -> ("Modbus master out"=w519:refnum<class "Modbus Master.lvclass">, "error out"=w518:errorcluster)
        n94 = Unbundle(w552) -> ("Modbus master out"=w524:refnum<class "Modbus Master.lvclass">, "error out"=w525:errorcluster)
        n95 = for {
          tunnel: w565 -> [w611] mode=indexing
          tunnel: [w610] -> w564 mode=indexing
          tunnel: [w609] -> w563 mode=indexing
          tunnel: [w608] -> w560 mode=indexing
          tunnel: [w599] -> w561 mode=indexing
          tunnel: [w607] -> w559 mode=indexing
          tunnel: [w603] -> w558 mode=indexing
          tunnel: [w602] -> w557 mode=indexing
          tunnel: [w606] -> w555 mode=indexing
          tunnel: [w605] -> w556 mode=indexing
          tunnel: [w604] -> w554 mode=indexing
          tunnel: [w601] -> w542 mode=indexing
          tunnel: [w600] -> w541 mode=indexing
          tunnel: [w597] -> w514 mode=indexing
          tunnel: w488 -> [w598] mode=indexing
          tunnel: [w596] -> w487 mode=indexing
          n96 = case shown="False" w598 {
            tunnel: w611 -> [w614 w652]
            tunnel: [w613 w647] -> w610
            tunnel: [w612 w646] -> w609
            tunnel: [w619 w638] -> w608
            tunnel: [w619 w637] -> w607
            tunnel: ["N/A" w636] -> w606
            tunnel: [FALSE w634] -> w605
            tunnel: [w619 w633] -> w604
            tunnel: [w619 w632] -> w603
            tunnel: [w619 w631] -> w602
            tunnel: [w620 w627] -> w601
            tunnel: [u16 1 ("register") w626] -> w600
            tunnel: [w619 w621] -> w596
            tunnel: [w620 w622] -> w599
            tunnel: [sgl 0.0 w621] -> w597
            frame False {
              w619 = sgl 0.0
              w620 = sgl[] [0.0, 0.0, 0.0]
              n97 = Unbundle(w614) -> ("Modbus master out"=w613:refnum<class "Modbus Master.lvclass">, "error out"=w612:errorcluster)
            }
            frame True {
              n98 = Unbundle(w652) -> ("Modbus master out"=w651:refnum<class "Modbus Master.lvclass">, "error out"=w650:errorcluster)
              n99 = call "Read_Electrical_Variables_v2.vi"("error in (no error)"=w650, "Modbus master in"=w651) -> ("error out"=w648:errorcluster, "Variables"=w643:sgl[], "Modbus master out"=w649:refnum<class "Modbus Master.lvclass">)  [unwired: 7 in]
              n100 = Index Array(array=w643, index #1=4, index #11=17 ("index")) -> (element #1=w625:sgl, element #2=w624:sgl, element #3=w623:sgl, element #4=w630:sgl, element #5=w629:sgl, element #6=w628:sgl, element #7=w621:sgl, element #8=w633:sgl, element #10=w638:sgl, element #11=w637:sgl, element #13=w632:sgl, element #14=w631:sgl)  [unwired: 12 in, 2 out]
              n101 = Build Array(w625, w624, w623) -> (w622:sgl[])
              n102 = Build Array(w630, w629, w628) -> (w627:sgl[])
              n103 = call "Read_Status.vi"("error in (no error)"=w648, "Modbus master in"=w649) -> ("error out"=w646:errorcluster, "Variables"=w641:u16[], "Modbus master out"=w647:refnum<class "Modbus Master.lvclass">)  [unwired: 7 in]
              n104 = Index Array(array=w641, index #3=3) -> (element #1=w626:u16, element #2=w640:u16, element #3=w639:u16)  [unwired: 2 in]
              n105 = case shown="0, Default" w639 {
                tunnel: ["Master Mode Simple" "Slave Mode Simple" "Master Mode Droops" "Slave Mode Droops"] -> w636
                frame 0, Default {
                }
                frame 1 {
                }
                frame 2 {
                }
                frame 3 {
                }
              }
              n106 = Number To Boolean Array(number=w640) -> (Boolean array=w635:bool[])
              n107 = Index Array(array=w635) -> (element=w634:bool)  [unwired: 1 in]
            }
          }
        }
        "ALL AC RMS Line-Line Average Voltage" <- w561
        "ALL Real Power" <- w487
        "ALL Reactive Power" <- w560
        "ALL State of Charge" <- w559
        "ALL Across Variable" <- w558
        "ALL Through Variable" <- w557
        "ALL Logged" <- w556
        "ALL Control Method" <- w555
        "ALL Frequency" <- w554
        "ALL AC RMS Line-Neutral Voltages" <- w542
        "ALL Status" <- w541
        n108 = case shown="No Error" w525 {
          selector: w525 -> [w584 w594]
          tunnel: w524 -> [w585 w595]
          tunnel: [w583 w587] -> w523
          tunnel: [w582 w595] -> w522
          tunnel: [w581 w594] -> w521
          tunnel: w519 -> [w579 w592]
          tunnel: w518 -> [w578 w589]
          tunnel: [w579 w591] -> w517
          tunnel: [w578 w590] -> w516
          tunnel: ["PQM" "Egauge"] -> w515
          tunnel: [sgl 60.0 w586] -> w492
          frame No Error {
            n109 = call "Read Electrical Variables ASCO PQM.vi"("Error in"=w584, "Modbus master in"=w585) -> ("Error out"=w581:errorcluster, "Electrical Variables"=w583:sgl[], "Modbus master out"=w582:refnum<class "Modbus Master.lvclass">)  [unwired: 7 in]
          }
          frame Error {
            n110 = call "Read Variables Egauge.vi"("error in (no error)"=w589, "Modbus master in"=w592) -> ("error out"=w590:errorcluster, "Variables"=w587:sgl[], "Modbus master out"=w591:refnum<class "Modbus Master.lvclass">)  [unwired: 7 in]
            n111 = Index Array(array=w587, index=11) -> (element=w586:sgl)
          }
        }
        "PCC Meter" <- w515
        "Frequency" <- w492
        n112 = for {
          tunnel: w502 -> [w576] mode=indexing
          tunnel: [w573] -> w501 mode=indexing
          tunnel: [w572] -> w500 mode=indexing
          tunnel: [w569] -> w498 mode=indexing
          n113 = Unbundle(w576) -> ("Modbus master out"=w575:refnum<class "Modbus Master.lvclass">, "error out"=w574:errorcluster)
          n114 = call "Read Variables Egauge.vi"("error in (no error)"=w574, "Modbus master in"=w575) -> ("error out"=w572:errorcluster, "Variables"=w571:sgl[], "Modbus master out"=w573:refnum<class "Modbus Master.lvclass">)  [unwired: 7 in]
          n115 = Index Array(array=w571, index=10) -> (element=w569:sgl)
        }
        "SOLAR Real Power" <- w498
        n116 = In Range and Coerce(upper limit=sgl 60.5, x=w492, lower limit=sgl 59.5) -> (In Range?=→"Correct":bool)  [unwired: 1 out]
        n117 = Index Array(array=w523, index #1=4 ("index"), index #4=10 ("index")) -> (element #1=w550:sgl, element #2=w549:sgl, element #3=w548:sgl, element #4=w538:sgl, element #5=→"PCC Frequency":sgl, element #7=→"PCC Reactive Power":sgl)  [unwired: 5 in, 1 out]
        "PCC Real Power" <- w538
        n118 = Compound Arithmetic op=ADD(w550, w549, w548) -> (w547:sgl)
        n119 = Bundle("Modbus master out"=w522, "error IO"=w521) -> (w520:T8)  [unwired: 1 in]
        n120 = Bundle("Modbus master out"=w517, "error out"=w516) -> (w526:T6)  [unwired: 1 in]
        n121 = Divide(x=w547, y=sgl 3.0) -> (x/y=→"PCC AC Line-Line Voltage":sgl)
        n122 = local write "SYS Status"("Reading") -> ()
        n123 = Add Array Elements(numeric array=w498) -> (sum=w497:sgl)
        n124 = Build Cluster Array(w501, w500) -> (w499:T5)
        n125 = Divide(x=w497, y=sgl 1000.0) -> (x/y=w493:sgl)
        "SOLAR Total Real Power" <- w493
        n126 = event shown="[12] \"DER8 Login Button\": Value Change" {
          selector: w535 -> [w657 _ _ _ w693 _ _ _ _ _ _ _ _ _ _ _ _ _ _ _ _ _ _ _ _]
          dyn-events: [w657 _ _ _ w693 _ _ _ _ _ _ _ _ _ _ _ _ _ _ _ _ _ _ _ _] -> w534
          timeout: 250 -> [_ _ _ _ _ _ _ _ _ _ _ _ _ _ _ _ _ _ _ _ _ _ _ _ _]
          tunnel: [1 w662 w673 w683 13 13 13 13 13 13 13 13 13 13 13 13 13 13 13 13 201 202 400 403 404] -> w567
          tunnel: [0 w661 w671 w682 0 1 2 3 4 5 6 7 8 9 10 11 12 13 14 15 ("DER") _ _ _ _ _] -> w553
          event Timeout {
            n127 = event-data() -> ()  [unwired: 1 in, 1 out]
          }
          event User Event {
            n128 = event-data() -> ("Asset"=w666:bool[])  [unwired: 1 in]
            n129 = Search 1D Array(1D array=w666, element=TRUE) -> (index of element=w660:i32)  [unwired: 1 in]
            n130 = Equal?(x=w660, y=-1) -> (x = y?=w663:bool)
            n131 = case shown="False" w663 {
              tunnel: [1000 0] -> w662
              tunnel: [w667 0 ("index of element")] -> w661
              tunnel: w660 -> [w667 _]
              frame False {
              }
              frame True {
              }
            }
          }
          event User Event {
            n132 = event-data() -> ("Command"=w674:bool[])  [unwired: 1 in]
            n133 = Boolean Array To Number(Boolean array=w674) -> (number=w675:u32)
            n134 = case shown="0, Default" w675 {
              tunnel: [0 11 12 14 15 500] -> w673
              frame 0, Default {
              }
              frame 1 {
              }
              frame 2 {
              }
              frame 4 {
              }
              frame 8 {
              }
              frame 16 {
              }
            }
            n135 = local read "data"() -> (w672:T1)
            n136 = Unbundle By Name(w672) -> ("DER"=w671:i32)
          }
          event User Event {
            n137 = event-data() -> ("Detail"=w687:bool[])  [unwired: 1 in]
            n138 = Search 1D Array(1D array=w687, element=TRUE) -> (index of element=w684:i32)  [unwired: 1 in]
            n139 = Equal?(x=w684, y=-1) -> (x = y?=w685:bool)
            n140 = case shown="False" w685 {
              tunnel: [1001 0] -> w683
              tunnel: [w689 0 ("index of element")] -> w682
              tunnel: w684 -> [w689 _]
              frame False {
              }
              frame True {
              }
            }
          }
          event "DER0 Login Button": Value Change {
            n141 = event-data() -> ()  [unwired: 1 in, 1 out]
          }
          event "DER1 Login Button": Value Change {
            n142 = event-data() -> ()  [unwired: 1 in, 1 out]
          }
          event "DER2 Login Button": Value Change {
            n143 = event-data() -> ()  [unwired: 1 in, 1 out]
          }
          event "DER3 Login Button": Value Change {
            n144 = event-data() -> ()  [unwired: 1 in, 1 out]
          }
          event "DER4 Login Button": Value Change {
            n145 = event-data() -> ()  [unwired: 1 in, 1 out]
          }
          event "DER5 Login Button": Value Change {
            n146 = event-data() -> ()  [unwired: 1 in, 1 out]
          }
          event "DER6 Login Button": Value Change {
            n147 = event-data() -> ()  [unwired: 1 in, 1 out]
          }
          event "DER7 Login Button": Value Change {
            n148 = event-data() -> ()  [unwired: 1 in, 1 out]
          }
          event "DER8 Login Button": Value Change {
            n149 = event-data() -> ()  [unwired: 1 in, 1 out]
          }
          event "DER9 Login Button": Value Change {
            n150 = event-data() -> ()  [unwired: 1 in, 1 out]
          }
          event "DER10 Login Button": Value Change {
            n151 = event-data() -> ()  [unwired: 1 in, 1 out]
          }
          event "DER11 Login Button": Value Change {
            n152 = event-data() -> ()  [unwired: 1 in, 1 out]
          }
          event "DER12 Login Button": Value Change {
            n153 = event-data() -> ()  [unwired: 1 in, 1 out]
          }
          event "DER13 Login Button": Value Change {
            n154 = event-data() -> ()  [unwired: 1 in, 1 out]
          }
          event "DER14 Login Button": Value Change {
            n155 = event-data() -> ()  [unwired: 1 in, 1 out]
          }
          event "DER15 Login Button": Value Change {
            n156 = event-data() -> ()  [unwired: 1 in, 6 out]
          }
          event "OPT Start Button": Value Change {
            n157 = event-data() -> ()  [unwired: 1 in, 1 out]
          }
          event "OPT Stop Button": Value Change {
            n158 = event-data() -> ()  [unwired: 1 in, 1 out]
          }
          event "Island": Value Change {
            n159 = event-data() -> ()  [unwired: 1 in, 1 out]
          }
          event "Relay 1": Value Change {
            n160 = event-data() -> ()  [unwired: 1 in, 1 out]
          }
          event "Relay 2": Value Change {
            n161 = event-data() -> ()  [unwired: 1 in, 6 out]
          }
        }
        n162 = Add Array Elements(numeric array=w514) -> (sum=w513:sgl)
        n163 = Divide(x=w513, y=sgl 1000.0) -> (x/y=w528:sgl)
        n164 = local read "OPT Microgrid Set-point"() -> (w504:sgl)
        n165 = Divide(x=w538, y=sgl 1000.0) -> (x/y=w530:sgl)
        "PCC Real Power Duplicate" <- w530
        n166 = Divide(x=w538, y=sgl 1000.0) -> (x/y=w512:sgl)
        n167 = local read "Pmax"() -> (w509:sgl)
        n168 = local read "Pmin"() -> (w506:sgl)
        n169 = Subtract(x=w530, y=w528) -> (x-y=w494:sgl)
        "Free Power Flow Gauge" <- w494
        "Free Power Flow Plot" <- w494
        "Free Power Flow" <- w494
        n170 = Divide(x=w509, y=w505) -> (x/y=w508:sgl)
        n171 = Divide(x=w506, y=w505) -> (x/y=w507:sgl)
        n172 = Build Array(w512, w494, w508, w507, w504) -> (w511:sgl[])
        n173 = Subtract(x=w494, y=w493) -> (x-y=→"LOAD Total Real Power":sgl)
        n174 = Array To Cluster(array=w511) -> (cluster=→"PCC Real Power Figure":T3)
        n175 = Build Cluster Array(w564, w563) -> (w562:T5)
        n176 = local write "SYS DER Index"(w553) -> ()
      }
      frame 1 {
        # "DER0: Heila 2 , CAPSTONE, .182\nDER1: Heila 4, AQUION, .184\nDER2: Heila 0, TESLA, .180\nDER3: Heila 22, Load Bank, .202\nDER4: Heila 9, MOTOR 1, .189\nDER5: Heila 8, SIMPLIPHI 1, .188\nDER6: Heila 10, GREEN SOLUTIONS, .190\nDER7: Heila 7, OUTBACK 1, .187\nDER8: Heila15, OUTBACK 2, .195\nDER9: Heila 12, SUNNY ISLAND, .191\nDER10: Heila 5, ESS, .185\nDER11: Heila 1, Fuel Cells, .181\nDER12: Heila 21. Sparkplug, .201\nDER13: Heila 12, Fronius, .192\nDER14: Heila 27, Sunny Boy, .207\nDER15: Heila 16, Motor 2, .196"
        n177 = local read "ALL AC RMS Line-Line Average Voltage"() -> (w745:sgl[][])
        n178 = local read "ALL Real Power"() -> (w744:sgl[])
        n179 = local read "ALL Frequency"() -> (w738:sgl[])
        n180 = local read "ALL Reactive Power"() -> (w743:sgl[])
        n181 = local read "ALL State of Charge"() -> (w742:sgl[])
        n182 = local read "ALL Across Variable"() -> (w737:sgl[])
        n183 = local read "ALL Through Variable"() -> (w736:sgl[])
        n184 = local read "ALL Status"() -> (w741:u16[])
        n185 = local read "ALL Logged"() -> (w740:bool[])
        n186 = local read "ALL Control Method"() -> (w739:string[])
        n187 = local read "ALL AC RMS Line-Neutral Voltages"() -> (w735:sgl[][])
        n188 = for {
          tunnel: w745 -> [w761] mode=indexing
          tunnel: w744 -> [w760] mode=indexing
          tunnel: w743 -> [w759] mode=indexing
          tunnel: w742 -> [w758] mode=indexing
          tunnel: w741 -> [w751] mode=indexing
          tunnel: w740 -> [w757] mode=indexing
          tunnel: w739 -> [w756] mode=indexing
          tunnel: w738 -> [w755] mode=indexing
          tunnel: w737 -> [w754] mode=indexing
          tunnel: w736 -> [w753] mode=indexing
          tunnel: w735 -> [w752] mode=indexing
          i -> [w762]
          n189 = case shown="1" w751 {
            tunnel: ["Operating" "OFF" "Sleeping" "Starting" "Stopping" "5: Busy" "6: N/A" "Fault" "Standby" "Generic Failure"] -> w750
            frame 0, Default {
            }
            frame 1 {
            }
            frame 2 {
            }
            frame 3 {
            }
            frame 4 {
            }
            frame 5 {
            }
            frame 6 {
            }
            frame 7 {
            }
            frame 8 {
            }
            frame 65535 {
            }
          }
          n190 = case shown="0, Default" w762 {
            tunnel: w761 -> [w780 w787 w802 w816 w827 w837 w848 w864 w878 w890 w901 w913 w921 w940 w956 w966]
            tunnel: w760 -> [w785 w797 w806 w817 w834 w844 w858 w871 w881 w894 w906 w912 w928 w944 w961 w971]
            tunnel: w759 -> [_ w793 w810 _ _ _ w854 _ _ _ _ _ _ w936 w953 _]
            tunnel: w758 -> [_ w800 w813 w818 w831 w845 w859 w861 w876 w888 w898 w911 w925 _ _ w969]
            tunnel: w757 -> [w786 w799 w814 w819 w836 w847 w860 w873 w883 w897 w908 w909 w931 w947 w964 w974]
            tunnel: w756 -> [w773 w798 w815 _ _ _ _ _ _ _ _ _ _ _ _ _]
            tunnel: w755 -> [_ _ w812 _ _ _ _ _ _ w885 _ _ _ _ _ _]
            tunnel: w754 -> [_ _ _ _ w835 w846 _ w872 w877 w887 w899 _ w930 _ w963 w973]
            tunnel: w753 -> [_ _ _ _ _ _ _ _ _ _ _ _ _ _ _ _]
            tunnel: w752 -> [_ _ _ _ _ _ _ _ w875 _ _ _ _ _ _ _]
            tunnel: w750 -> [w774 w791 w801 w820 w826 w841 w852 w868 w879 w893 w904 w910 w926 w946 w962 w975]
            frame 0, Default {
              n191 = Add Array Elements(numeric array=w780) -> (sum=w783:sgl)
              n192 = Divide(x=w785, y=sgl 1000.0) -> (x/y=w779:sgl)
              "DER0 Real Power" <- w779
              n193 = Divide(x=w783, y=3.0) -> (x/y=→"DER0 AC Line-Line Voltage":dbl)
              n194 = Divide(x=w779, y=sgl 65.0) -> (x/y=w777:sgl)
              n195 = Multiply(x=w777, y=sgl 100.0) -> (x*y=→"DER0 Power Level" →"DER0 Power Level Figure":sgl)
              "DER0 Logged" <- w786
              "DER0 State" <- w774
              "Indicator 0" <- w780
              "DER0 Control Mode" <- w773
            }
            frame 1 {
              n196 = Add Array Elements(numeric array=w787) -> (sum=w790:sgl)
              n197 = Divide(x=w790, y=3.0) -> (x/y=→"DER1 AC Line-Line Voltage":dbl)
              n198 = Divide(x=w793, y=sgl 1000.0) -> (x/y=→"DER1 Reactive Power":sgl)
              n199 = Divide(x=w797, y=sgl 1000.0) -> (x/y=→"DER1 Real Power":sgl)
              "DER1 State of Charge" <- w800
              "DER1 State of Charge Figure" <- w800
              "DER1 Logged" <- w799
              "DER1 Control Mode" <- w798
              "DER1 State" <- w791
              "Indicator 1" <- w787
            }
            frame 2 {
              n200 = Add Array Elements(numeric array=w802) -> (sum=w805:sgl)
              n201 = Divide(x=w805, y=3.0) -> (x/y=→"DER2 AC Line-Line Voltage":dbl)
              n202 = Divide(x=w810, y=sgl 1000.0) -> (x/y=→"DER2 Reactive Power":sgl)
              n203 = Divide(x=w806, y=sgl 1000.0) -> (x/y=→"DER2 Real Power":sgl)
              "DER2 Logged" <- w814
              "DER2 Control Mode" <- w815
              "DER2 Frequency" <- w812
              "DER2 State of Charge" <- w813
              "DER2 State of Charge Figure" <- w813
              "DER2 State" <- w801
              "Indicator 2" <- w802
            }
            frame 3 {
              n204 = Divide(x=w817, y=1000.0) -> (x/y=→"DER3 Real Power":dbl)
              n205 = Add Array Elements(numeric array=w816) -> (sum=w825:sgl)
              n206 = Divide(x=w825, y=3.0) -> (x/y=→"DER3 AC Line-Line Votlage":dbl)
              "DER3 Logged" <- w819
              "DER3 State" <- w820
              "Indicator 3" <- w816
              "DER3 State of Charge" <- w818
              "DER3 State of Charge Figure" <- w818
            }
            frame 4 {
              n207 = Add Array Elements(numeric array=w827) -> (sum=w830:sgl)
              n208 = Divide(x=w834, y=sgl 1000.0) -> (x/y=→"DER4 Real Power":sgl)
              n209 = Divide(x=w830, y=3.0) -> (x/y=→"DER4 AC Line-Line Votlage":dbl)
              "DER4 State of Charge" <- w831
              "DER4 State of Charge Figure" <- w831
              "DER4 Logged" <- w836
              "DER4 Across Variable" <- w835
              "DER4 State" <- w826
              "Indicator 4" <- w827
            }
            frame 5 {
              n210 = Divide(x=w844, y=sgl 1000.0) -> (x/y=→"DER5 Real Power":sgl)
              n211 = Add Array Elements(numeric array=w837) -> (sum=w840:sgl)
              n212 = Divide(x=w840, y=1.0) -> (x/y=→"DER5 AC Line-Line Votlage":dbl)
              "DER5 Across Variable" <- w846
              "DER5 logged" <- w847
              "DER5 State of Charge Figure" <- w845
              "DER5 State of Charge" <- w845
              "DER5 State" <- w841
              "Indicator 5" <- w837
            }
            frame 6 {
              n213 = Add Array Elements(numeric array=w848) -> (sum=w851:sgl)
              n214 = Divide(x=w858, y=sgl 1000.0) -> (x/y=→"DER6 Real Power":sgl)
              n215 = Divide(x=w854, y=sgl 1000.0) -> (x/y=→"DER6 Reactive Power":sgl)
              n216 = Divide(x=w851, y=1.0) -> (x/y=→"DER6 AC Line-Line Voltage":dbl)
              "DER Logged" <- w860
              "DER6 State of Charge" <- w859
              "DER6 State of Charge Figure" <- w859
              "DER6 State" <- w852
              "Indicator 6" <- w848
            }
            frame 7 {
              n217 = Add Array Elements(numeric array=w864) -> (sum=w867:sgl)
              n218 = Divide(x=w861, y=sgl 1.0) -> (x/y=→"DER7 State of Charge" →"DER7 State of Charge Figure":sgl)
              n219 = Divide(x=w871, y=sgl 1000.0) -> (x/y=→"DER7 Real Power":sgl)
              n220 = Divide(x=w867, y=3.0) -> (x/y=→"DER7 AC Line-Line Voltage":dbl)
              "DER7 DC Voltage" <- w872
              "DER7 Logged" <- w873
              "DER7 State" <- w868
              "Indicator 7" <- w864
            }
            frame 8 {
              n221 = Index Array(array=w875) -> (element=→"DER8 AC Line-Line Votlage":sgl)  [unwired: 1 in]
              n222 = Divide(x=w881, y=sgl 1000.0) -> (x/y=→"DER8 Real Power":sgl)
              "DER8 Logged" <- w883
              "DER8 State" <- w879
              "Indicator 8" <- w878
              "DER8 DC Voltage" <- w877
              "DER8 State of Charge Figure" <- w876
              "DER8 State of Charge" <- w876
            }
            frame 9 {
              n223 = Add Array Elements(numeric array=w890) -> (sum=w892:sgl)
              n224 = Divide(x=w892, y=3.0) -> (x/y=→"DER9 AC Line-Line Votlage":dbl)
              n225 = Divide(x=w885, y=sgl 1000.0) -> (x/y=→"DER9 Reactive Power":sgl)
              n226 = Divide(x=w894, y=sgl 1000.0) -> (x/y=→"DER9 Real Power":sgl)
              "DER9 Logged" <- w897
              "DER9 State" <- w893
              "Indicator 9" <- w890
              "DER9 Across Variable" <- w887
              "DER9 State of Charge Figure" <- w888
              "DER9 State of Charge" <- w888
            }
            frame 10 {
              n227 = Add Array Elements(numeric array=w901) -> (sum=w903:sgl)
              n228 = Divide(x=w906, y=sgl 1000.0) -> (x/y=→"DER10 Real Power":sgl)
              n229 = Divide(x=w903, y=3.0) -> (x/y=→"DER10 AC Line-Line Votlage":dbl)
              "DER10 Logged" <- w908
              "DER10 State" <- w904
              "Indicator 10" <- w901
              "DER10 DC Voltage" <- w899
              "DER10 State of Charge" <- w898
              "DER10 State of Charge Figure" <- w898
            }
            frame 11 {
              n230 = Divide(x=w912, y=sgl 1000.0) -> (x/y=→"DER11 Real Power":sgl)
              n231 = Divide(x=w912, y=sgl 1000.0) -> (x/y=→"DER11 Reactive Power":sgl)
              n232 = Add Array Elements(numeric array=w913) -> (sum=w918:sgl)
              n233 = Divide(x=w918, y=3.0) -> (x/y=→"DER11 AC Line-Line Votlage":dbl)
              "DER11 Logged" <- w909
              "DER11 State" <- w910
              "Indicator 11" <- w913
              "DER11 State of Charge" <- w911
              "DER11 State of Charge Figure" <- w911
            }
            frame 12 {
              n234 = Add Array Elements(numeric array=w921) -> (sum=w924:sgl)
              n235 = Divide(x=w928, y=sgl 1000.0) -> (x/y=→"DER12 Real Power":sgl)
              n236 = Divide(x=w924, y=1.0) -> (x/y=→"DER12 AC Line-Line Votlage":dbl)
              "DER12 Logged" <- w931
              "DER12 DC Voltage" <- w930
              "DER12 State" <- w926
              "DER12 State of Charge Figure" <- w925
              "DER12 State of Charge" <- w925
              "Indicator 12" <- w921
            }
            frame 13 {
              n237 = Add Array Elements(numeric array=w940) -> (sum=w943:sgl)
              n238 = Divide(x=w944, y=sgl 1000.0) -> (x/y=w935:sgl)
              "DER13 Real Power" <- w935
              n239 = Divide(x=w936, y=sgl 1000.0) -> (x/y=→"DER13 Reactive Power":sgl)
              n240 = Divide(x=w943, y=1.0) -> (x/y=→"DER13 AC Line-Line Voltage":dbl)
              n241 = Divide(x=w935, y=sgl 2.0) -> (x/y=w933:sgl)
              n242 = Multiply(x=w933, y=sgl 100.0) -> (x*y=→"DER13 Power Level Figure" →"DER13 Power Level":sgl)
              "DER13 Logged" <- w947
              "DER13 State" <- w946
              "Indicator 13" <- w940
            }
            frame 14 {
              n243 = Add Array Elements(numeric array=w956) -> (sum=w959:sgl)
              n244 = Divide(x=w961, y=sgl 1000.0) -> (x/y=w952:sgl)
              "DER14 Real Power" <- w952
              n245 = Divide(x=w953, y=sgl 1000.0) -> (x/y=→"DER14 Reactive Power":sgl)
              n246 = Divide(x=w959, y=1.0) -> (x/y=→"DER14 AC Line-Line Voltage":dbl)
              n247 = Divide(x=w952, y=sgl 3.0) -> (x/y=w950:sgl)
              n248 = Multiply(x=w950, y=sgl 100.0) -> (x*y=→"DER14 Power Level Figure" →"DER14 Power Level":sgl)
              "DER14 DC Voltage" <- w963
              "DER14 Logged" <- w964
              "DER14 State" <- w962
              "Indicator 14" <- w956
            }
            frame 15 {
              n249 = Add Array Elements(numeric array=w966) -> (sum=w968:sgl)
              n250 = Divide(x=w971, y=sgl 1000.0) -> (x/y=→"DER15 Real Power":sgl)
              n251 = Divide(x=w968, y=3.0) -> (x/y=→"DER15 AC Line-Line Voltage":dbl)
              "DER15 DC Voltage" <- w973
              "DER15 State" <- w975
              "DER15 Logged" <- w974
              "DER15 State of Charge" <- w969
              "DER15 State of Charge Figure" <- w969
              "Indicator 15" <- w966
            }
          }
        }
        n252 = local write "SYS Status"("Processing" ("Status")) -> ()
        n253 = Wait Until Next ms Multiple(millisecond multiple=u32 250) -> ()  [unwired: 1 out]
      }
      frame 2 {
        n254 = local read "PCC AC Line-Line Voltage"() -> (w995:sgl)
        n255 = local read "PCC Reactive Power"() -> (w997:sgl)
        n256 = local read "ALL State of Charge"() -> (w977:sgl[])
        n257 = local read "ALL Reactive Power"() -> (w984:sgl[])
        n258 = local read "PCC Real Power"() -> (w998:sgl)
        n259 = local read "PCC Frequency"() -> (w996:sgl)
        n260 = local read "ALL Real Power"() -> (w988:sgl[])
        n261 = local read "SYS Current Time"() -> (w979:dbl)
        n262 = local read "ALL Frequency"() -> (w983:sgl[])
        n263 = local read "SOLAR Real Power"() -> (w976:sgl[])
        n264 = local write "SYS Status"("Saving" ("Status")) -> ()
        n265 = Build Array (concatenate)(w979, w998, w997, w996, w995, w988, w984, w983, w977, w976) -> (w987:dbl[])
        n266 = Reshape Array(w987, 75 ("dimension size")) -> (w986:dbl[])
        n267 = local read "OPT Optimization Running Indicator"() -> (w1003:bool)
        n268 = Array To Spreadsheet String(array=w986, 3:"%f" ("format string")) -> (spreadsheet string=w993:string)  [unwired: 1 in]
        n269 = case shown="True" w1003 {
          tunnel: [w1005 200] -> w1002
          tunnel: 0 -> [w1005 _]
          frame False {
          }
          frame True {
          }
        }
        n270 = Write to Text File(file (use dialog)=w990, text=w993, error in=w989) -> (refnum out=w992:refnum<file>, error out=w991:errorcluster)  [unwired: 1 in, 1 out]
        n271 = Wait Until Next ms Multiple(millisecond multiple=u32 250) -> ()  [unwired: 1 out]
      }
      frame 11 {
        n272 = local read "SYS DER Index"() -> (w1010:i32)
        n273 = Index Array(array=w1014, index=w1010) -> (element=w1019:T6)
        n274 = Unbundle(w1019) -> ("Modbus master out"=w1018:refnum<class "Modbus Master.lvclass">, "error out"=w1017:errorcluster)
        n275 = local write "SYS Status"("Start" ("Status")) -> ()
        n276 = call-dynamic "Write Single Holding Register.vi"("error in (no error)"=w1017, "holding register value"=u16 1, "address"=u16 2032 ("starting address"), "Modbus master in"=w1018) -> ("error out"=w1015:errorcluster, "Modbus master out"=w1016:refnum<class "Modbus Master.lvclass">)  [unwired: 6 in]
        n277 = Bundle("Modbus master out"=w1016, "error out"=w1015) -> (w1013:T6)  [unwired: 1 in]
        n278 = Wait Until Next ms Multiple(millisecond multiple=u32 250) -> ()  [unwired: 1 out]
        n279 = Replace Array Subset(array=w1014, new element=w1013, index=w1010) -> (w1012:T5)
      }
      frame 12 {
        n280 = local read "SYS DER Index"() -> (w1028:i32)
        n281 = Index Array(array=w1030, index=w1028) -> (element=w1036:T6)
        n282 = Unbundle(w1036) -> ("Modbus master out"=w1035:refnum<class "Modbus Master.lvclass">, "error out"=w1034:errorcluster)
        n283 = local write "SYS Status"("Stop" ("Status")) -> ()
        n284 = call-dynamic "Write Single Holding Register.vi"("error in (no error)"=w1034, "holding register value"=u16 0, "address"=u16 2032 ("starting address"), "Modbus master in"=w1035) -> ("error out"=w1032:errorcluster, "Modbus master out"=w1033:refnum<class "Modbus Master.lvclass">)  [unwired: 6 in]
        n285 = Bundle("Modbus master out"=w1033, "error out"=w1032) -> (w1031:T6)  [unwired: 1 in]
        n286 = Replace Array Subset(array=w1030, new element=w1031, index=w1028) -> (w1029:T5)
        n287 = Wait Until Next ms Multiple(millisecond multiple=u32 250) -> ()  [unwired: 1 out]
      }
      frame 13 {
        n288 = local read "SYS DER Index"() -> (w1044:i32)
        n289 = String To Byte Array(string="HEILA") -> (unsigned byte array=w1059:u8[])
        n290 = Index Array(array=w1053, index=w1044) -> (element=w1055:T6)
        n291 = for {
          N: 16 -> [_]
          tunnel: w1059 -> [w1070]
          tunnel: [w1069] -> w1047 mode=indexing
          i -> [w1065]
          n292 = Multiply(x=w1065, y=2) -> (x*y=w1066:i32)
          n293 = Increment(x=w1066) -> (x+1=w1067:i32)
          n294 = Index Array(array=w1070, index #1=w1066, index #2=w1067) -> (element #1=w1064:u8, element #2=w1062:u8)
          n295 = To Unsigned Byte Integer(number=w1064) -> (unsigned 8bit integer=w1063:u8)
          n296 = To Unsigned Byte Integer(number=w1062) -> (unsigned 8bit integer=w1061:u8)
          n297 = Join Numbers(hi=w1063, lo=w1061) -> ((hi.lo)=w1069:u16)
        }
        n298 = Unbundle(w1055) -> ("Modbus master out"=w1048:refnum<class "Modbus Master.lvclass">, "error out"=w1054:errorcluster)
        n299 = call-dynamic "Write Multiple Holding Registers.vi"("error in (no error)"=w1054, "holding register values"=w1047, "starting address"=u16 2000, "Modbus master in"=w1048) -> ("error out"=w1051:errorcluster, "Modbus master out"=w1052:refnum<class "Modbus Master.lvclass">)  [unwired: 6 in]
        n300 = local write "SYS Status"("Login" ("Status")) -> ()
        n301 = Bundle("Modbus master out"=w1052, "error out"=w1051) -> (w1050:T6)  [unwired: 1 in]
        n302 = Replace Array Subset(array=w1053, new element=w1050, index=w1044) -> (w1049:T5)
        n303 = Wait Until Next ms Multiple(millisecond multiple=u32 250) -> ()  [unwired: 1 out]
      }
      frame 14 {
        n304 = local read "SYS DER Index"() -> (w1077:i32)
        n305 = Index Array(array=w1086, index=w1077) -> (element=w1087:T6)
        n306 = local read "data"() -> (w1074:T1)
        n307 = Unbundle By Name(w1074) -> ("Variable 1 Setpoint"=w1075:sgl)
        n308 = Type Cast(type=u32 0, x=w1075) -> (*(type *) &x=w1092:u32)
        n309 = Split Number(x=w1092) -> (hi(x)=w1090:u16, lo(x)=w1089:u16)
        n310 = Unbundle(w1087) -> ("Modbus master out"=w1084:refnum<class "Modbus Master.lvclass">, "error out"=w1083:errorcluster)
        n311 = Build Array(w1090, w1089) -> (w1078:u16[])
        n312 = call-dynamic "Write Multiple Holding Registers.vi"("error in (no error)"=w1083, "holding register values"=w1078, "starting address"=u16 2036, "Modbus master in"=w1084) -> ("error out"=w1081:errorcluster, "Modbus master out"=w1082:refnum<class "Modbus Master.lvclass">)  [unwired: 6 in]
        n313 = local write "SYS Status"("Set Real Power" ("Status")) -> ()
        n314 = Bundle("Modbus master out"=w1082, "error out"=w1081) -> (w1080:T6)  [unwired: 1 in]
        n315 = Replace Array Subset(array=w1086, new element=w1080, index=w1077) -> (w1085:T5)
        n316 = Wait Until Next ms Multiple(millisecond multiple=u32 10) -> ()  [unwired: 1 out]
      }
      frame 15 {
        n317 = local read "SYS DER Index"() -> (w1099:i32)
        n318 = local read "data"() -> (w1098:T1)
        n319 = Index Array(array=w1100, index=w1099) -> (element=w1109:T6)
        n320 = Unbundle By Name(w1098) -> ("Variable 2 Setpoint"=w1097:sgl)
        n321 = Type Cast(type=u32 0, x=w1097) -> (*(type *) &x=w1113:u32)
        n322 = Split Number(x=w1113) -> (hi(x)=w1111:u16, lo(x)=w1110:u16)
        n323 = Unbundle(w1109) -> ("Modbus master out"=w1108:refnum<class "Modbus Master.lvclass">, "error out"=w1107:errorcluster)
        n324 = Build Array(w1111, w1110) -> (w1102:u16[])
        n325 = call-dynamic "Write Multiple Holding Registers.vi"("error in (no error)"=w1107, "holding register values"=w1102, "starting address"=u16 2038, "Modbus master in"=w1108) -> ("error out"=w1105:errorcluster, "Modbus master out"=w1106:refnum<class "Modbus Master.lvclass">)  [unwired: 6 in]
        n326 = Bundle("Modbus master out"=w1106, "error out"=w1105) -> (w1104:T6)  [unwired: 1 in]
        n327 = Replace Array Subset(array=w1100, new element=w1104, index=w1099) -> (w1101:T5)
        n328 = Wait Until Next ms Multiple(millisecond multiple=u32 50) -> ()  [unwired: 1 out]
      }
      frame 16 {
        # "V"
        n329 = local read "SYS DER Index"() -> (w1121:i32)
        n330 = local read "data"() -> (w1120:T1)
        n331 = Index Array(array=w1123, index=w1121) -> (element=w1131:T6)
        n332 = Unbundle By Name(w1120) -> ("Variable 1 Setpoint"=w1119:sgl)
        n333 = Type Cast(type=u32 0, x=w1119) -> (*(type *) &x=w1135:u32)
        n334 = Split Number(x=w1135) -> (hi(x)=w1133:u16, lo(x)=w1132:u16)
        n335 = Unbundle(w1131) -> ("Modbus master out"=w1130:refnum<class "Modbus Master.lvclass">, "error out"=w1129:errorcluster)
        n336 = Build Array(w1133, w1132) -> (w1124:u16[])
        n337 = call-dynamic "Write Multiple Holding Registers.vi"("error in (no error)"=w1129, "holding register values"=w1124, "starting address"=u16 2040, "Modbus master in"=w1130) -> ("error out"=w1127:errorcluster, "Modbus master out"=w1128:refnum<class "Modbus Master.lvclass">)  [unwired: 6 in]
        n338 = Bundle("Modbus master out"=w1128, "error out"=w1127) -> (w1126:T6)  [unwired: 1 in]
        n339 = Replace Array Subset(array=w1123, new element=w1126, index=w1121) -> (w1122:T5)
        n340 = Wait Until Next ms Multiple(millisecond multiple=u32 50) -> ()  [unwired: 1 out]
      }
      frame 17 {
        n341 = local read "SYS DER Index"() -> (w1143:i32)
        n342 = local read "data"() -> (w1142:T1)
        n343 = Index Array(array=w1145, index=w1143) -> (element=w1153:T6)
        n344 = Unbundle By Name(w1142) -> ("Variable 2 Setpoint"=w1141:sgl)
        n345 = Type Cast(type=u32 0, x=w1141) -> (*(type *) &x=w1157:u32)
        n346 = Split Number(x=w1157) -> (hi(x)=w1155:u16, lo(x)=w1154:u16)
        n347 = Unbundle(w1153) -> ("Modbus master out"=w1152:refnum<class "Modbus Master.lvclass">, "error out"=w1151:errorcluster)
        n348 = Build Array(w1155, w1154) -> (w1146:u16[])
        n349 = call-dynamic "Write Multiple Holding Registers.vi"("error in (no error)"=w1151, "holding register values"=w1146, "starting address"=u16 2042, "Modbus master in"=w1152) -> ("error out"=w1149:errorcluster, "Modbus master out"=w1150:refnum<class "Modbus Master.lvclass">)  [unwired: 6 in]
        n350 = Bundle("Modbus master out"=w1150, "error out"=w1149) -> (w1148:T6)  [unwired: 1 in]
        n351 = Replace Array Subset(array=w1145, new element=w1148, index=w1143) -> (w1144:T5)
        n352 = Wait Until Next ms Multiple(millisecond multiple=u32 250) -> ()  [unwired: 1 out]
      }
      frame 200 {
        n353 = local read "OPT Microgrid Set-point"() -> (w1167:sgl)
        n354 = local read "PCC Real Power"() -> (w1184:sgl)
        n355 = local read "OPT Alpha"() -> (w1185:sgl)
        n356 = local read "OPT Price"() -> (w1186:sgl[])
        n357 = Multiply(x=w1167, y=sgl 1000.0) -> (x*y=w1166:sgl)
        n358 = Subtract(x=w1166, y=w1184) -> (x-y=w1191:sgl)
        n359 = Multiply(x=w1191, y=w1185) -> (x*y=w1190:sgl)
        n360 = Index Array(array=w1186) -> (element=w1189:sgl)  [unwired: 1 in]
        n361 = Add(x=w1190, y=w1189) -> (x+y=w1188:sgl)
        n362 = local read "Free Power Flow Plot"() -> (w1175:sgl)
        n363 = Build Array(w1188, w1188, w1188, w1188, w1188) -> (w1187:sgl[])
        n364 = case shown="True" "Reset Dual Variables" {
          tunnel: [w1200 sgl[] [0.0, 0.0, 0.0, 0.0, 0.0]] -> w1183
          tunnel: w1187 -> [w1200 _]
          frame False {
          }
          frame True {
          }
        }
        n365 = for {
          tunnel: w1195 -> [w1214] mode=indexing
          tunnel: w1183 -> [w1211]
          tunnel: [w1207] -> w1182 mode=indexing
          tunnel: [w1205] -> w1181 mode=indexing
          tunnel: [w1204] -> w1179 mode=indexing
          tunnel: [w1203] -> w1178 mode=indexing
          tunnel: "Array DER Index Dispatch" -> [w1202] mode=indexing
          n366 = Unbundle(w1214) -> ("Modbus master out"=w1213:refnum<class "Modbus Master.lvclass">, "error out"=w1212:errorcluster)
          n367 = call "Heila IQ Optimization.vi"("Index"=w1202, "error in (no error)"=w1212, "Dispatch"="Dispatch", "Price"=w1211, "Modbus master in"=w1213) -> ("error out"=w1208:errorcluster, "Output Variables"=w1210:sgl[], "Modbus master out"=w1209:refnum<class "Modbus Master.lvclass">)  [unwired: 4 in]
          n368 = Index Array(array=w1210) -> (element #1=w1205:sgl, element #2=w1204:sgl, element #3=w1203:sgl)  [unwired: 3 in]
          n369 = Bundle("Modbus master out"=w1209, "error out"=w1208) -> (w1207:T6)  [unwired: 1 in]
        }
        "Bid" <- w1181
        "Pmax,i" <- w1179
        "Pmin,i" <- w1178
        n370 = Multiply(x=w1175, y=sgl 1000.0) -> (x*y=w1173:sgl)
        n371 = Add Array Elements(numeric array=w1179) -> (sum=w1180:sgl)
        n372 = Add Array Elements(numeric array=w1178) -> (sum=w1172:sgl)
        n373 = local read "OPT Microgrid Set-point"() -> (w1170:sgl)
        n374 = local write "OPT Price"(w1183) -> ()
        n375 = Add(x=w1173, y=w1180) -> (x+y=w1176:sgl)
        "Pmax" <- w1176
        n376 = Add(x=w1173, y=w1172) -> (x+y=w1171:sgl)
        "Pmin" <- w1171
        n377 = Multiply(x=w1170, y=sgl 1000.0) -> (x*y=w1169:sgl)
        n378 = In Range and Coerce(upper limit=w1176, x=w1169, lower limit=w1171) -> (coerced(x)=w1162:sgl, In Range?=→"In Range?":bool)
        n379 = Wait Until Next ms Multiple(millisecond multiple=250) -> ()  [unwired: 1 out]
        n380 = case shown="True" "Coerce" {
          tunnel: w1162 -> [_ w1197]
          frame False {
          }
          frame True {
            n381 = Divide(x=w1197, y=sgl 1000.0) -> (x/y=w1199:sgl)
            n382 = local write "OPT Microgrid Set-point"(w1199) -> ()
          }
        }
      }
      frame 201 {
        # "Start Optimization"
        n383 = for {
          tunnel: w1223 -> [w1231] mode=indexing
          tunnel: [w1226] -> w1222 mode=indexing
          tunnel: [w1225] -> w1221 mode=indexing
          n384 = Unbundle(w1231) -> ("Modbus master out"=w1230:refnum<class "Modbus Master.lvclass">, "error out"=w1229:errorcluster)
          n385 = call-dynamic "Write Single Holding Register.vi"("error in (no error)"=w1229, "holding register value"=u16 1, "address"=u16 5000, "Modbus master in"=w1230) -> ("error out"=w1225:errorcluster, "Modbus master out"=w1226:refnum<class "Modbus Master.lvclass">)  [unwired: 6 in]
        }
        n386 = Build Cluster Array(w1222, w1221) -> (w1220:T5)
        n387 = local write "OPT Optimization Running Indicator"(TRUE ("Optimization Running")) -> ()
        n388 = Wait Until Next ms Multiple(millisecond multiple=u32 100) -> ()  [unwired: 1 out]
      }
      frame 202 {
        # "Stop optimization"
        n389 = for {
          tunnel: w1237 -> [w1248] mode=indexing
          tunnel: [w1243] -> w1239 mode=indexing
          tunnel: [w1242] -> w1238 mode=indexing
          n390 = Unbundle(w1248) -> ("Modbus master out"=w1247:refnum<class "Modbus Master.lvclass">, "error out"=w1246:errorcluster)
          n391 = call-dynamic "Write Single Holding Register.vi"("error in (no error)"=w1246, "holding register value"=u16 0, "address"=u16 5000, "Modbus master in"=w1247) -> ("error out"=w1242:errorcluster, "Modbus master out"=w1243:refnum<class "Modbus Master.lvclass">)  [unwired: 6 in]
        }
        n392 = Build Cluster Array(w1239, w1238) -> (w1236:T5)
        n393 = local write "OPT Optimization Running Indicator"(FALSE ("Optimization Running")) -> ()
        n394 = Wait Until Next ms Multiple(millisecond multiple=u32 100) -> ()  [unwired: 1 out]
      }
      frame 400 {
        n395 = Unbundle(w1258) -> ("Modbus master out"=w1257:refnum<class "Modbus Master.lvclass">, "error out"=w1256:errorcluster)
        n396 = flat-sequence {
          tunnel: w1257 -> [w1263]
          tunnel: w1256 -> [w1262]
          tunnel: [w1266] -> w1255
          tunnel: [w1265] -> w1254
          tunnel: w1255 -> [w1272]
          tunnel: w1254 -> [w1271]
          tunnel: [w1270] -> w1253
          tunnel: [w1269] -> w1252
          frame #0 {
            n397 = call-dynamic "Write Single Holding Register.vi"("error in (no error)"=w1262, "holding register value"=u16 12345, "address"=u16 998, "Modbus master in"=w1263) -> ("error out"=w1265:errorcluster, "Modbus master out"=w1266:refnum<class "Modbus Master.lvclass">)  [unwired: 6 in]
            n398 = Wait Until Next ms Multiple(millisecond multiple=u32 250) -> ()  [unwired: 1 out]
          }
          frame #1 {
            n399 = call-dynamic "Write Single Holding Register.vi"("error in (no error)"=w1271, "holding register value"=u16 0, "address"=u16 4140, "Modbus master in"=w1272) -> ("error out"=w1269:errorcluster, "Modbus master out"=w1270:refnum<class "Modbus Master.lvclass">)  [unwired: 6 in]
          }
        }
        n400 = Bundle("Modbus master out"=w1253, "error out"=w1252) -> (w1251:T6)  [unwired: 1 in]
        n401 = Wait Until Next ms Multiple(millisecond multiple=u32 250) -> ()  [unwired: 1 out]
      }
      frame 403 {
        n402 = Unbundle(w1284) -> ("Modbus master out"=w1283:refnum<class "Modbus Master.lvclass">, "error out"=w1282:errorcluster)
        n403 = flat-sequence {
          tunnel: w1283 -> [w1289]
          tunnel: w1282 -> [w1288]
          tunnel: [w1292] -> w1281
          tunnel: [w1291] -> w1280
          tunnel: w1281 -> [w1299]
          tunnel: w1280 -> [w1298]
          tunnel: [w1297] -> w1279
          tunnel: [w1296] -> w1278
          frame #0 {
            n404 = call-dynamic "Write Single Holding Register.vi"("error in (no error)"=w1288, "holding register value"=u16 12345, "address"=u16 998, "Modbus master in"=w1289) -> ("error out"=w1291:errorcluster, "Modbus master out"=w1292:refnum<class "Modbus Master.lvclass">)  [unwired: 6 in]
            n405 = Wait Until Next ms Multiple(millisecond multiple=u32 250) -> ()  [unwired: 1 out]
          }
          frame #1 {
            n406 = call-dynamic "Write Single Holding Register.vi"("error in (no error)"=w1298, "holding register value"="Relay 1 Num", "address"=u16 4139, "Modbus master in"=w1299) -> ("error out"=w1296:errorcluster, "Modbus master out"=w1297:refnum<class "Modbus Master.lvclass">)  [unwired: 6 in]
          }
        }
        n407 = Bundle("Modbus master out"=w1279, "error out"=w1278) -> (w1277:T6)  [unwired: 1 in]
        n408 = Wait Until Next ms Multiple(millisecond multiple=u32 250) -> ()  [unwired: 1 out]
      }
      frame 404 {
        n409 = Unbundle(w1310) -> ("Modbus master out"=w1309:refnum<class "Modbus Master.lvclass">, "error out"=w1308:errorcluster)
        n410 = flat-sequence {
          tunnel: w1309 -> [w1315]
          tunnel: w1308 -> [w1314]
          tunnel: [w1318] -> w1307
          tunnel: [w1317] -> w1306
          tunnel: w1307 -> [w1325]
          tunnel: w1306 -> [w1324]
          tunnel: [w1323] -> w1305
          tunnel: [w1322] -> w1304
          frame #0 {
            n411 = call-dynamic "Write Single Holding Register.vi"("error in (no error)"=w1314, "holding register value"=u16 12345, "address"=u16 998, "Modbus master in"=w1315) -> ("error out"=w1317:errorcluster, "Modbus master out"=w1318:refnum<class "Modbus Master.lvclass">)  [unwired: 6 in]
            n412 = Wait Until Next ms Multiple(millisecond multiple=u32 250) -> ()  [unwired: 1 out]
          }
          frame #1 {
            n413 = call-dynamic "Write Single Holding Register.vi"("error in (no error)"=w1324, "holding register value"="Relay 2 Num", "address"=u16 4140, "Modbus master in"=w1325) -> ("error out"=w1322:errorcluster, "Modbus master out"=w1323:refnum<class "Modbus Master.lvclass">)  [unwired: 6 in]
          }
        }
        n414 = Bundle("Modbus master out"=w1305, "error out"=w1304) -> (w1303:T6)  [unwired: 1 in]
        n415 = Wait Until Next ms Multiple(millisecond multiple=u32 250) -> ()  [unwired: 1 out]
      }
      frame 401 {
        n416 = Unbundle(w1336) -> ("Modbus master out"=w1335:refnum<class "Modbus Master.lvclass">, "error out"=w1334:errorcluster)
        n417 = flat-sequence {
          tunnel: w1335 -> [w1341]
          tunnel: w1334 -> [w1340]
          tunnel: [w1344] -> w1333
          tunnel: [w1343] -> w1332
          tunnel: w1333 -> [w1350]
          tunnel: w1332 -> [w1349]
          tunnel: [w1348] -> w1331
          tunnel: [w1347] -> w1330
          frame #0 {
            n418 = call-dynamic "Write Single Holding Register.vi"("error in (no error)"=w1340, "holding register value"=u16 12345, "address"=u16 998, "Modbus master in"=w1341) -> ("error out"=w1343:errorcluster, "Modbus master out"=w1344:refnum<class "Modbus Master.lvclass">)  [unwired: 6 in]
            n419 = Wait Until Next ms Multiple(millisecond multiple=u32 250) -> ()  [unwired: 1 out]
          }
          frame #1 {
            n420 = call-dynamic "Write Single Holding Register.vi"("error in (no error)"=w1349, "holding register value"=u16 0, "address"=u16 4139, "Modbus master in"=w1350) -> ("error out"=w1347:errorcluster, "Modbus master out"=w1348:refnum<class "Modbus Master.lvclass">)  [unwired: 6 in]
          }
        }
        n421 = Bundle("Modbus master out"=w1331, "error out"=w1330) -> (w1329:T6)  [unwired: 1 in]
        n422 = Wait Until Next ms Multiple(millisecond multiple=u32 250) -> ()  [unwired: 1 out]
      }
      frame 402 {
        n423 = Unbundle(w1368) -> ("Modbus master out"=w1367:refnum<class "Modbus Master.lvclass">, "error out"=w1366:errorcluster)
        n424 = flat-sequence {
          tunnel: w1367 -> [w1373]
          tunnel: w1366 -> [w1372]
          tunnel: [w1376] -> w1365
          tunnel: [w1375] -> w1364
          tunnel: w1365 -> [w1382]
          tunnel: w1364 -> [w1381]
          tunnel: [w1380] -> w1363
          tunnel: [w1379] -> w1362
          tunnel: w1363 -> [w1387]
          tunnel: w1362 -> [w1386]
          tunnel: [w1387] -> w1361
          tunnel: [w1386] -> w1360
          tunnel: w1361 -> [w1392]
          tunnel: w1360 -> [w1391]
          tunnel: [w1389] -> w1359
          tunnel: [w1388] -> w1358
          tunnel: w1359 -> [w1399]
          tunnel: w1358 -> [w1398]
          tunnel: [w1396] -> w1357
          tunnel: [w1395] -> w1356
          frame #0 {
            n425 = call-dynamic "Write Single Holding Register.vi"("error in (no error)"=w1372, "holding register value"=u16 12345, "address"=u16 998, "Modbus master in"=w1373) -> ("error out"=w1375:errorcluster, "Modbus master out"=w1376:refnum<class "Modbus Master.lvclass">)  [unwired: 6 in]
            n426 = Wait Until Next ms Multiple(millisecond multiple=u32 250) -> ()  [unwired: 1 out]
          }
          frame #1 {
            n427 = call-dynamic "Write Single Holding Register.vi"("error in (no error)"=w1381, "holding register value"=u16 1, "address"=u16 4140, "Modbus master in"=w1382) -> ("error out"=w1379:errorcluster, "Modbus master out"=w1380:refnum<class "Modbus Master.lvclass">)  [unwired: 6 in]
          }
          frame #2 {
            n428 = Wait Until Next ms Multiple(millisecond multiple=u32 1000) -> ()  [unwired: 1 out]
          }
          frame #3 {
            n429 = Wait Until Next ms Multiple(millisecond multiple=u32 250) -> ()  [unwired: 1 out]
            n430 = call-dynamic "Write Single Holding Register.vi"("error in (no error)"=w1391, "holding register value"=u16 12345, "address"=u16 998, "Modbus master in"=w1392) -> ("error out"=w1388:errorcluster, "Modbus master out"=w1389:refnum<class "Modbus Master.lvclass">)  [unwired: 6 in]
          }
          frame #4 {
            n431 = call-dynamic "Write Single Holding Register.vi"("error in (no error)"=w1398, "holding register value"=u16 1, "address"=u16 4139, "Modbus master in"=w1399) -> ("error out"=w1395:errorcluster, "Modbus master out"=w1396:refnum<class "Modbus Master.lvclass">)  [unwired: 6 in]
          }
        }
        n432 = Wait Until Next ms Multiple(millisecond multiple=u32 250) -> ()  [unwired: 1 out]
        n433 = Bundle("Modbus master out"=w1357, "error out"=w1356) -> (w1355:T6)  [unwired: 1 in]
      }
      frame 500 {
        n434 = local read "data"() -> (w1406:T1)
        n435 = local read "SYS DER Index"() -> (w1402:i32)
        n436 = Unbundle By Name(w1406) -> ("Cotrol Mode"=w1405:enum16{"Master", "Slave"})
        n437 = Index Array(array=w1408, index=w1402) -> (element=w1412:T6)
        n438 = case shown="\"Master\"" w1405 {
          tunnel: [u16 0 ("holding register value") u16 1 ("holding register value")] -> w1416
          frame "Master" {
          }
          frame "Slave", Default {
          }
        }
        n439 = Unbundle(w1412) -> ("Modbus master out"=w1414:refnum<class "Modbus Master.lvclass">, "error out"=w1413:errorcluster)
        n440 = call-dynamic "Write Single Holding Register.vi"("error in (no error)"=w1413, "holding register value"=w1416, "address"=u16 2035, "Modbus master in"=w1414) -> ("error out"=w1410:errorcluster, "Modbus master out"=w1411:refnum<class "Modbus Master.lvclass">)  [unwired: 6 in]
        n441 = Bundle("Modbus master out"=w1411, "error out"=w1410) -> (w1409:T6)  [unwired: 1 in]
        n442 = Replace Array Subset(array=w1408, new element=w1409, index=w1402) -> (w1407:T5)
      }
      frame 1000 {
        n443 = property class="VI"(reference=w1424) -> ("Exec.State"=w1425:T9)  [unwired: 1 in, 2 out]
        n444 = case shown="\"Idle\"" w1425 {
          tunnel: w1426 -> [_ w1440 _ _]
          tunnel: w1424 -> [_ w1430 w1449 w1451]
          tunnel: [0 0 1000 1000] -> w1423
          frame "Bad", Default {
          }
          frame "Idle" {
            n445 = invoke class="VI" method="Run VI"(reference=w1430, "Wait until done"=FALSE ("Wait Until Done"), "Auto Dispose Ref"=FALSE ("Auto Dispose Reference")) -> (reference out=w1436:refnum<vi>)  [unwired: 2 in, 4 out]
            n446 = local read "SYS DER Index"() -> (w1443:i32)
            n447 = invoke class="VI" method="FP.Open"(reference=w1436, "Activate"=TRUE ("Activate?"), "State"=T7."Standard") -> (reference out=w1435:refnum<vi>)  [unwired: 2 in, 4 out]
            n448 = To Variant(anything=w1443) -> (Variant=w1445:variant)
            n449 = invoke class="VI" method="Ctrl Val.Set"(reference=w1435, "Control Name"="DER", "Value"=w1445) -> (reference out=w1441:refnum<vi>)  [unwired: 2 in, 4 out]
            n450 = To Variant(anything=w1440) -> (Variant=w1442:variant)
            n451 = invoke class="VI" method="Ctrl Val.Set"(reference=w1441, "Control Name"="Event", "Value"=w1442) -> (reference out=w1432:refnum<vi>)  [unwired: 2 in, 4 out]
            n452 = To Variant(anything="DER List") -> (Variant=w1434:variant)
            n453 = invoke class="VI" method="Ctrl Val.Set"(reference=w1432, "Control Name"="DER Names", "Value"=w1434) -> ()  [unwired: 2 in, 5 out]
          }
          frame "Run top level" {
            n454 = invoke class="VI" method="Abort VI"(reference=w1449) -> ()  [unwired: 2 in, 3 out]
          }
          frame "Running" {
            n455 = invoke class="VI" method="Abort VI"(reference=w1451) -> ()  [unwired: 2 in, 3 out]
          }
        }
      }
      frame 1001 {
        n456 = property class="VI"(reference=w1452) -> ("Exec.State"=w1457:T9)  [unwired: 1 in, 2 out]
        n457 = case shown="\"Idle\"" w1457 {
          tunnel: w1452 -> [_ w1466 w1476 w1478]
          tunnel: [0 0 1000 1000] -> w1456
          frame "Bad", Default {
          }
          frame "Idle" {
            n458 = invoke class="VI" method="Run VI"(reference=w1466, "Wait until done"=FALSE ("Wait Until Done"), "Auto Dispose Ref"=FALSE ("Auto Dispose Reference")) -> (reference out=w1462:refnum<vi>)  [unwired: 2 in, 4 out]
            n459 = local read "SYS DER Index"() -> (w1472:i32)
            n460 = invoke class="VI" method="FP.Open"(reference=w1462, "Activate"=TRUE ("Activate?"), "State"=T7."Standard") -> (reference out=w1463:refnum<vi>)  [unwired: 2 in, 4 out]
            n461 = To Variant(anything=w1472) -> (Variant=w1474:variant)
            n462 = invoke class="VI" method="Ctrl Val.Set"(reference=w1463, "Control Name"="DER", "Value"=w1474) -> (reference out=w1467:refnum<vi>)  [unwired: 2 in, 4 out]
            n463 = local read "DER List"() -> (w1468:string[])
            n464 = To Variant(anything=w1468) -> (Variant=w1470:variant)
            n465 = invoke class="VI" method="Ctrl Val.Set"(reference=w1467, "Control Name"="DER Names", "Value"=w1470) -> ()  [unwired: 2 in, 5 out]
          }
          frame "Run top level" {
            n466 = invoke class="VI" method="Abort VI"(reference=w1476) -> ()  [unwired: 2 in, 3 out]
          }
          frame "Running" {
            n467 = invoke class="VI" method="Abort VI"(reference=w1478) -> ()  [unwired: 2 in, 3 out]
          }
        }
      }
    }
    n468 = local read "ALL Real Power"() -> (w205:sgl[])
    n469 = for {
      tunnel: w205 -> [w287] mode=indexing
      i -> [w292]
      n470 = Greater?(x=w287, y=sgl 200.0) -> (0:w300:bool)
      n471 = Less?(x=w287, y=sgl -200.0) -> (x < y?=w299:bool)
      n472 = Greater?(x=w287, y=sgl 1000.0) -> (0:w286:bool)
      n473 = Less?(x=w287, y=sgl -1000.0) -> (x < y?=w285:bool)
      n474 = Greater?(x=w287, y=sgl 5000.0) -> (0:w284:bool)
      n475 = Less?(x=w287, y=sgl -5000.0) -> (x < y?=w283:bool)
      n476 = Build Array(w300, w299, w286, w285, w284, w283) -> (w298:bool[])
      n477 = local read "SYS Iteration"() -> (w294:i32)
      n478 = Boolean Array To Number(Boolean array=w298) -> (number=w296:u32)
      n479 = Quotient & Remainder(x=w294, y=3) -> (x-y*floor(x/y)=w293:i32)  [unwired: 1 out]
      n480 = case shown="42" w296 {
        tunnel: [0 ("x") w307 w333 w360 w387 w415 w443] -> w297
        tunnel: w293 -> [_ w305 w332 w358 w385 w413 w441]
        tunnel: w292 -> [_ w304 w330 w361 w389 w417 w445]
        frame 0, Default {
        }
        frame 1 {
          # "> 500W"
          n481 = case shown="0, Default" w304 {
            tunnel: [1 ("x") 1 ("x") 4 ("x") 1 ("x") 1 ("x") 4 ("x") 1 ("x") 1 ("x") 4 ("x") 4 ("x") 4 ("x") 4 ("x") 4 ("x") 4 ("x") 1 ("x") 1 ("x") 4 ("x") 4 ("x") 1 ("x") 1 ("x") 1 ("x") 1 ("x")] -> w306
            frame 0, Default {
            }
            frame 1 {
            }
            frame 2 {
            }
            frame 3 {
            }
            frame 4 {
            }
            frame 5 {
            }
            frame 6 {
            }
            frame 7 {
            }
            frame 8 {
            }
            frame 9 {
            }
            frame 10 {
            }
            frame 11 {
            }
            frame 12 {
            }
            frame 13 {
            }
            frame 14 {
            }
            frame 15 {
            }
            frame 16 {
            }
            frame 17 {
            }
            frame 18 {
            }
            frame 19 {
            }
            frame 20 {
            }
            frame 21 {
            }
          }
          n482 = Add(x=w306, y=w305) -> (x+y=w307:i32)
        }
        frame 2 {
          # "< -500W"
          n483 = case shown="0, Default" w330 {
            tunnel: [4 ("x") 4 ("x") 1 ("x") 4 ("x") 4 ("x") 1 ("x") 4 ("x") 4 ("x") 1 ("x") 1 ("x") 1 ("x") 1 ("x") 1 ("x") 1 ("x") 4 ("x") 4 ("x") 1 ("x") 1 ("x") 4 ("x") 4 ("x") 4 ("x") 4 ("x")] -> w331
            frame 0, Default {
            }
            frame 1 {
            }
            frame 2 {
            }
            frame 3 {
            }
            frame 4 {
            }
            frame 5 {
            }
            frame 6 {
            }
            frame 7 {
            }
            frame 8 {
            }
            frame 9 {
            }
            frame 10 {
            }
            frame 11 {
            }
            frame 12 {
            }
            frame 13 {
            }
            frame 14 {
            }
            frame 15 {
            }
            frame 16 {
            }
            frame 17 {
            }
            frame 18 {
            }
            frame 19 {
            }
            frame 20 {
            }
            frame 21 {
            }
          }
          n484 = Add(x=w331, y=w332) -> (x+y=w333:i32)
        }
        frame 5 {
          # "> 2000W"
          n485 = case shown="0, Default" w361 {
            tunnel: [1 ("x") 1 ("x") 4 ("x") 1 ("x") 1 ("x") 4 ("x") 1 ("x") 1 ("x") 4 ("x") 4 ("x") 4 ("x") 4 ("x") 4 ("x") 4 ("x") 1 ("x") 1 ("x") 4 ("x") 4 ("x") 1 ("x") 1 ("x") 1 ("x") 1 ("x")] -> w359
            frame 0, Default {
            }
            frame 1 {
            }
            frame 2 {
            }
            frame 3 {
            }
            frame 4 {
            }
            frame 5 {
            }
            frame 6 {
            }
            frame 7 {
            }
            frame 8 {
            }
            frame 9 {
            }
            frame 10 {
            }
            frame 11 {
            }
            frame 12 {
            }
            frame 13 {
            }
            frame 14 {
            }
            frame 15 {
            }
            frame 16 {
            }
            frame 17 {
            }
            frame 18 {
            }
            frame 19 {
            }
            frame 20 {
            }
            frame 21 {
            }
          }
          n486 = Add(x=6, y=w358) -> (x+y=w356:i32)
          n487 = Add(x=w359, y=w356) -> (x+y=w360:i32)
        }
        frame 10 {
          # "< -2000W"
          n488 = case shown="0, Default" w389 {
            tunnel: [4 ("x") 4 ("x") 1 ("x") 4 ("x") 4 ("x") 1 ("x") 4 ("x") 4 ("x") 1 ("x") 1 ("x") 1 ("x") 1 ("x") 1 ("x") 1 ("x") 4 ("x") 4 ("x") 1 ("x") 1 ("x") 4 ("x") 4 ("x") 4 ("x") 4 ("x")] -> w388
            frame 0, Default {
            }
            frame 1 {
            }
            frame 2 {
            }
            frame 3 {
            }
            frame 4 {
            }
            frame 5 {
            }
            frame 6 {
            }
            frame 7 {
            }
            frame 8 {
            }
            frame 9 {
            }
            frame 10 {
            }
            frame 11 {
            }
            frame 12 {
            }
            frame 13 {
            }
            frame 14 {
            }
            frame 15 {
            }
            frame 16 {
            }
            frame 17 {
            }
            frame 18 {
            }
            frame 19 {
            }
            frame 20 {
            }
            frame 21 {
            }
          }
          n489 = Add(x=6, y=w385) -> (x+y=w384:i32)
          n490 = Add(x=w388, y=w384) -> (x+y=w387:i32)
        }
        frame 21 {
          # "> 8000W"
          n491 = case shown="0, Default" w417 {
            tunnel: [1 ("x") 1 ("x") 4 ("x") 1 ("x") 1 ("x") 4 ("x") 1 ("x") 1 ("x") 4 ("x") 4 ("x") 4 ("x") 4 ("x") 4 ("x") 4 ("x") 1 ("x") 1 ("x") 4 ("x") 4 ("x") 1 ("x") 1 ("x") 1 ("x") 1 ("x")] -> w416
            frame 0, Default {
            }
            frame 1 {
            }
            frame 2 {
            }
            frame 3 {
            }
            frame 4 {
            }
            frame 5 {
            }
            frame 6 {
            }
            frame 7 {
            }
            frame 8 {
            }
            frame 9 {
            }
            frame 10 {
            }
            frame 11 {
            }
            frame 12 {
            }
            frame 13 {
            }
            frame 14 {
            }
            frame 15 {
            }
            frame 16 {
            }
            frame 17 {
            }
            frame 18 {
            }
            frame 19 {
            }
            frame 20 {
            }
            frame 21 {
            }
          }
          n492 = Add(x=12, y=w413) -> (x+y=w412:i32)
          n493 = Add(x=w416, y=w412) -> (x+y=w415:i32)
        }
        frame 42 {
          # "< -8000W"
          n494 = case shown="3" w445 {
            tunnel: [4 ("x") 4 ("x") 1 ("x") 4 ("x") 4 ("x") 1 ("x") 4 ("x") 4 ("x") 1 ("x") 1 ("x") 1 ("x") 1 ("x") 1 ("x") 1 ("x") 4 ("x") 4 ("x") 1 ("x") 1 ("x") 4 ("x") 4 ("x") 4 ("x") 4 ("x")] -> w444
            frame 0, Default {
            }
            frame 1 {
            }
            frame 2 {
            }
            frame 3 {
            }
            frame 4 {
            }
            frame 5 {
            }
            frame 6 {
            }
            frame 7 {
            }
            frame 8 {
            }
            frame 9 {
            }
            frame 10 {
            }
            frame 11 {
            }
            frame 12 {
            }
            frame 13 {
            }
            frame 14 {
            }
            frame 15 {
            }
            frame 16 {
            }
            frame 17 {
            }
            frame 18 {
            }
            frame 19 {
            }
            frame 20 {
            }
            frame 21 {
            }
          }
          n495 = Add(x=12, y=w441) -> (x+y=w440:i32)
          n496 = Add(x=w444, y=w440) -> (x+y=w443:i32)
        }
      }
      n497 = case shown="11" w292 {
        tunnel: w297 -> [w468 w469 w470 _ w472 w473 w474 w475 w476 w477 w478 _ w480 w481 w482 _ _ _ w483 _ _ _]
        frame 0, Default {
          "DER0 Flow" <- w468
        }
        frame 1 {
          "DER1 Flow" <- w469
        }
        frame 2 {
          "DER2 Flow" <- w470
        }
        frame 3 {
          "DER3 Flow" <- 0 ("DER3 Flow")
        }
        frame 4 {
          "DER4 Flow" <- w472
        }
        frame 5 {
          "DER5 Flow" <- w473
        }
        frame 6 {
          "DER6 Flow" <- w474
        }
        frame 7 {
          "DER7 Flow" <- w475
        }
        frame 8 {
          "DER8 Flow" <- w476
        }
        frame 9 {
          "DER9 Flow" <- w477
        }
        frame 10 {
          "DER10 Flow" <- w478
        }
        frame 11 {
          "DER11 Flow" <- 0 ("DER11 Flow")
        }
        frame 12 {
          "DER12 Flow" <- w480
        }
        frame 13 {
          "DER13 Flow" <- w481
        }
        frame 14 {
          "DER14 Flow" <- w482
        }
        frame 19 {
        }
        frame 20 {
        }
        frame 21 {
        }
        frame 15 {
          "DER15 Flow" <- w483
        }
        frame 16 {
        }
        frame 17 {
        }
        frame 18 {
        }
      }
    }
    n498 = local read "SOLAR Total Real Power"() -> (w115:sgl)
    n499 = local read "LOAD Total Real Power"() -> (w109:sgl)
    n500 = Negate(x=w109) -> (-x=w110:sgl)
    n501 = Build Array(w115, w110) -> (w114:sgl[])
    n502 = for {
      tunnel: [w221] -> w113 mode=indexing
      tunnel: w114 -> [w218] mode=indexing
      n503 = Multiply(x=w218, y=sgl 1000.0) -> (x*y=w219:sgl)
      n504 = local read "SYS Iteration"() -> (w220:i32)
      n505 = Greater?(x=w219, y=sgl 1500.0) -> (0:w232:bool)
      n506 = Less?(x=w219, y=sgl -1500.0) -> (x < y?=w231:bool)
      n507 = Greater?(x=w219, y=sgl 5000.0) -> (0:w226:bool)
      n508 = Less?(x=w219, y=sgl -5000.0) -> (x < y?=w225:bool)
      n509 = Greater?(x=w219, y=sgl 10000.0) -> (0:w224:bool)
      n510 = Less?(x=w219, y=sgl -10000.0) -> (x < y?=w223:bool)
      n511 = Build Array(w232, w231, w226, w225, w224, w223) -> (w222:bool[])
      n512 = Quotient & Remainder(x=w220, y=3) -> (x-y*floor(x/y)=w236:i32)  [unwired: 1 out]
      n513 = Boolean Array To Number(Boolean array=w222) -> (number=w235:u32)
      n514 = case shown="21" w235 {
        tunnel: [0 w240 w243 w246 w249 w252 w255] -> w221
        tunnel: w236 -> [_ w239 w242 w245 w248 w251 w254]
        frame 0, Default {
        }
        frame 1 {
          n515 = Add(x=1, y=w239) -> (x+y=w240:i32)
        }
        frame 2 {
          n516 = Add(x=4, y=w242) -> (x+y=w243:i32)
        }
        frame 5 {
          n517 = Add(x=7, y=w245) -> (x+y=w246:i32)
        }
        frame 10 {
          n518 = Add(x=10, y=w248) -> (x+y=w249:i32)
        }
        frame 21 {
          n519 = Add(x=13, y=w251) -> (x+y=w252:i32)
        }
        frame 42 {
          n520 = Add(x=16, y=w254) -> (x+y=w255:i32)
        }
      }
    }
    n521 = local write "SYS Case"(w168) -> ()
    n522 = Unbundle(w214) -> ("Modbus master out"=w162:refnum<class "Modbus Master.lvclass">, "error out"=w159:errorcluster)
    "PQM Current Error" <- w159
    n523 = Unbundle(w166) -> ("Modbus master out"=w165:refnum<class "Modbus Master.lvclass">, "error out"=w158:errorcluster)
    "Egauge Current Error" <- w158
    n524 = for {
      tunnel: w212 -> [w486] mode=indexing
      tunnel: [w485] -> w211 mode=indexing
      tunnel: [w486] -> w209 mode=indexing
      tunnel: [w484] -> w210 mode=indexing
      n525 = Unbundle(w486) -> ("error out"=w485:errorcluster)  [unwired: 1 out]
      n526 = Unbundle By Name(w485) -> ("status"=w484:bool)
    }
    "ALL DER Current Error" <- w211
    "ALL Error Indicator" <- w210
    n527 = Unbundle By Name(w159) -> ("status"=w157:bool)
    n528 = Unbundle By Name(w158) -> ("status"=w156:bool)
    n529 = for {
      tunnel: w154 -> [w261] mode=indexing
      tunnel: [w260] -> _ mode=indexing
      tunnel: [w261] -> _ mode=indexing
      tunnel: [w259] -> w153 mode=indexing
      n530 = Unbundle(w261) -> ("error out"=w260:errorcluster)  [unwired: 1 out]
      n531 = Unbundle By Name(w260) -> ("status"=w259:bool)
    }
    "Solar Meter Error Indicators" <- w153
    n532 = Build Array(w157, w156) -> (→"PCC Meter Error Indicators":bool[])
    n533 = Index Array(array=w113) -> (element #1=→"SOLAR Flow":i32, element #2=→"LOAD Flow":i32)  [unwired: 2 in]
    n534 = Bundle("Modbus master out"=w165, "error out"=w158) -> (w164:T6)  [unwired: 1 in]
    n535 = Bundle("Modbus master out"=w162, "error out"=w159) -> (w161:T6)  [unwired: 1 in]
  }
  n536 = Unbundle(w17) -> ("Modbus master out"=w16:refnum<class "Modbus Master.lvclass">, "error out"=w15:errorcluster)
  n537 = Unbundle(w20) -> ("Modbus master out"=w22:refnum<class "Modbus Master.lvclass">, "error out"=w21:errorcluster)
  n538 = Close File(refnum=w48, error in=w47) -> (error out=→"error out 3":errorcluster)  [unwired: 1 out]
  n539 = for {
    tunnel: w67 -> [w1482] mode=indexing
    tunnel: [w1479] -> w73 mode=indexing
    n540 = Unbundle(w1482) -> ("Modbus master out"=w1481:refnum<class "Modbus Master.lvclass">, "error out"=w1480:errorcluster)
    n541 = call-dynamic "Close.vi"("error in (no error)"=w1480, "Modbus master in"=w1481) -> ("error out"=w1479:errorcluster)  [unwired: 9 in]
  }
  "ALL DER Final Error" <- w73
  n542 = for {
    tunnel: w6 -> [w1486] mode=indexing
    tunnel: [w1483] -> w5 mode=indexing
    n543 = Unbundle(w1486) -> ("Modbus master out"=w1485:refnum<class "Modbus Master.lvclass">, "error out"=w1484:errorcluster)
    n544 = call-dynamic "Close.vi"("error in (no error)"=w1484, "Modbus master in"=w1485) -> ("error out"=w1483:errorcluster)  [unwired: 9 in]
  }
  "Array" <- w5
  n545 = call-dynamic "Close.vi"("error in (no error)"=w15, "Modbus master in"=w16) -> ("error out"=→"PQM Final Error":errorcluster)  [unwired: 9 in]
  n546 = call-dynamic "Close.vi"("error in (no error)"=w21, "Modbus master in"=w22) -> ("error out"=→"Egauge Final Error":errorcluster)  [unwired: 9 in]
  n547 = Unregister For Events(event registration refnum=w35) -> ()  [unwired: 1 in, 1 out]
  n548 = Destroy User Event(user event=w34) -> ()  [unwired: 1 in, 1 out]
  n549 = Destroy User Event(user event=w31) -> ()  [unwired: 1 in, 1 out]
  "SYS Iteration" <- 0
  "OPT Optimization Running Indicator" <- FALSE
  "SYS DER Index" <- 0 ("DER Index")
  "SYS Status" <- "Initializing" ("Sys Status")
  "SYS Case" <- 0 ("SYS Case")
  "Attempts" <- 0
  "OPT Running No Error" <- TRUE ("Boolean")
